vi "002_Data Source Manage.vi"(11 "Queue Ref In":T1={"UI"=refnum, "Message"=refnum, "Data"=refnum, "Caller"=refnum, "Name"="000 Common", "Data Path"=path "", "Class Path"=path "", "SubPanel"=refnum, "Project Name"="", "MNT"="", "Title"="", "Data Source"=refnum, "Queue List"={}, "VI"=refnum, "UE"=refnum}) -> ()   [LabVIEW 2020]
uses:
  Alin/QMH/000 Module Data Type.ctl
  Alin/QMH/Queue Message.ctl
  0007 Controls/002 Group Type.ctl
  0007 Controls/005 Data Source Type.ctl
  9999 SubVI/Global/Data Global/SDQ Data Type.ctl
  9999 SubVI/Global/Data Global/Data Global Mode.ctl
  <vilib>/Utility/file.llb/Read Delimited Spreadsheet (string).vi
  <vilib>/Utility/file.llb/Write Delimited Spreadsheet (string).vi
  <vilib>/Utility/config.llb/Write Key (String).vi
  <vilib>/Utility/config.llb/NI_LVConfig.lvlib
panel:
  in  "Module Launch":bool
  in  "Panel Show":bool
  in  "Data Source List":string(tree)
  out "Count":string
  in  "CAN Convert":bool
  in  "Show Info":bool
  in  "LabVIEW VISA":bool
  in  "SIEMENS S7":bool
  in  "FCTS DAQ":bool
  in  "Log List":i32(listbox)
  out "Write Time":u32(graph)
  out "Log":string
  out "Time":string
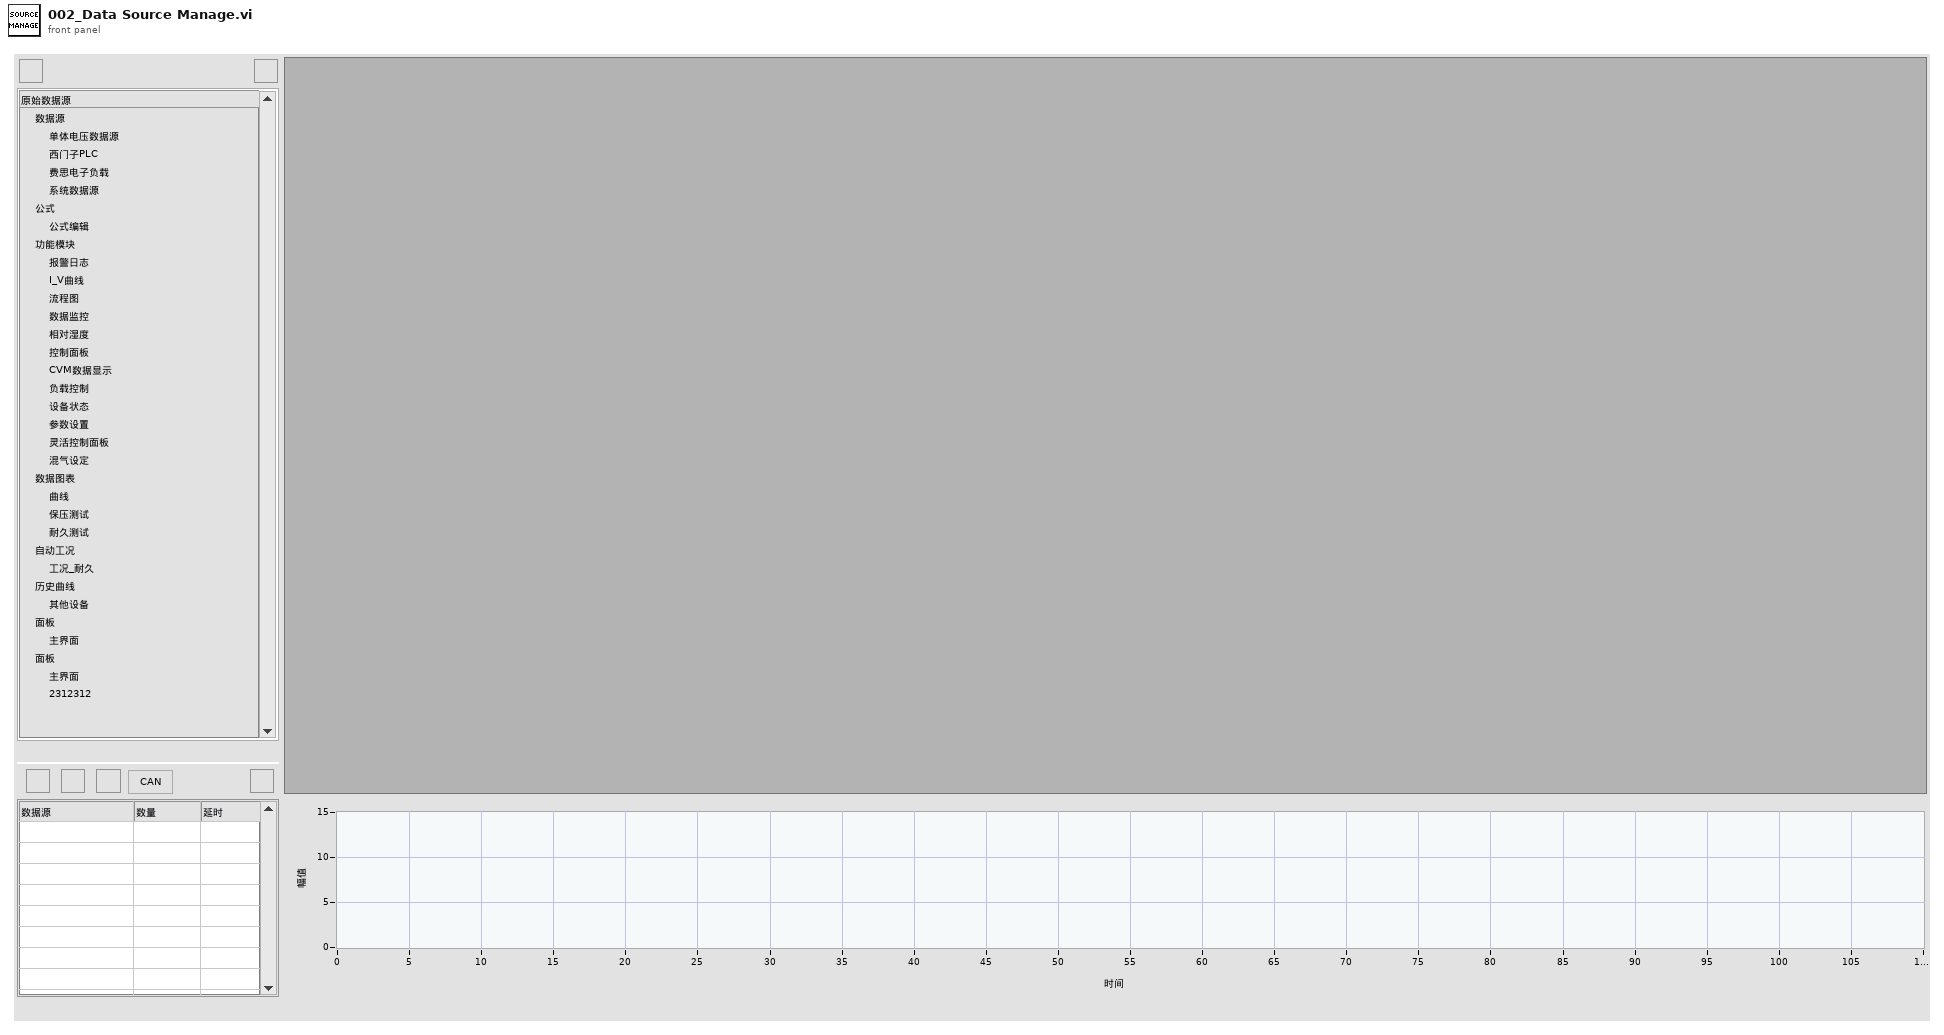
[diagram p1: front panel]
types:
  T1 = typedef "000 Module Data Type.ctl" = cluster{"UI":refnum<queue>, "Message":refnum<queue>, "Data":refnum<queue>, "Caller":refnum<queue>, "Name":string, "Data Path":path, "Class Path":path, "SubPanel":refnum<vi>, "Project Name":string, "MNT":string, "Title":string, "Data Source":refnum<queue>, "Queue List":map{string, refnum<queue>}, "VI":refnum<vi>, "UE":refnum<user-event>}
  T2 = typedef "SDQ Data Type.ctl" = cluster{"CAN Length":string, "CAN Name":string, "CAN ID":string, "CAN Type":string, "Test Item":string, "Byte Order":string, "Instruction":string, "Control Type":string, "Group":string, "Offset":dbl, "Coefficient":dbl, "Write Enable":bool, "Lable Type":string, "Key?":string, "Set Value":string, "Upper":dbl, "Lower":dbl, "Unit":string, "Formula":string, "Test Item Type":string, "Length":i32, "Address":string, "Name":string, "Identifier":string, "Data Type":string, "Enumerate?":string, "Enumerate List":string, "Data":string, "Source":string}
  T3 = cluster{"Queue":T1, "Source":map{string, map{string, T2}}, "All Data":map{string, T2}, "Type":cluster{"Name":string, "Data":map{string, T2}}, "Write Source":map{string, map{string, string}}, "Type":map{string, string}, "Log List":refnum<vi>, "Log":string[][], "Delay":cluster{"Count Time(ms)":u32, "Delay Time(ms)":u32, "Next":string}, "Internal?":bool, "Log Nane":string, "DataType":cluster{"Name":string, "Type":map{string, string}}, "DataMonitor":string[], "LoadControl":string}
  T4 = enum32{"Invalid", "Standard", "Closed", "Hidden", "Minimized", "Maximized"}
  T5 = typedef "Data Global Mode.ctl" = enum16{"Init", "Read", "Write", "Write Data", "Load"}
  T6 = cluster{"Name":string, "Type":map{string, string}}
  T7 = typedef "eventvkey.ctl" = enum16{"ASCII", "Enter", "Return", "Shift", "Ctrl", "Alt", "Cmd", "Opt", "Caps", "NumLock", "Clear", "Break", "Up", "Down", "Left", "Right", "Insert", "Delete", "Home", "End", "PageUp", "PageDown", "Escape", "Help", "Pause", "ScrollLock", "F1", "F2", "F3", "F4", "F5", "F6", "F7", "F8", "F9", "F10", "F11", "F12", "F13", "F14", "F15", "F16", "F17", "F18", "F19", "F20", "F21", "F22", "F23", "F24", "Play", "VolumeUp", "VolumeDown", "Mute", "Two Byte Char"}
  T8 = cluster{"Shift":bool, "Ctrl":bool, "Alt":bool, "Cmd":bool, "Opt":bool}
  T9 = typedef "002 Group Type.ctl" = cluster{"Name":string, "Enable":string, "Path":string}
  T10 = typedef "005 Data Source Type.ctl" = cluster{"Device Name":string, "Device Model":string, "Device Driver":string, "IP Address":string, "Port":string, "Remark":string, "Enable":string, "Path":string}
  T11 = cluster{"Queue":T1, "Data Source List":refnum<vi>, "SubPanel":refnum<vi>, "Group":cluster{"Group Title":string[], "Group Data":T9, "Group Name":string[]}, "Source":cluster{"Source Title":string[], "Source Data":T10, "Source Name":string[]}, "All Panel":string[], "GroupInfo":map{string, cluster{"Source":map{string, T10}, "Group":T9}}, "Class":map{string, cluster{"Device_Type":string, "Device_Manufacturer":string, "Driver":string, "Device_Model":string, "Class Path":path, "Defaule Config Path":string}}, "Version Path":path, "Source Launch?":bool, "Launch":bool}
  T12 = map{string, cluster{"Device_Type":string, "Device_Manufacturer":string, "Driver":string, "Device_Model":string, "Class Path":path, "Defaule Config Path":string}}
  T13 = cluster{"Device_Type":string, "Device_Manufacturer":string, "Driver":string, "Device_Model":string, "Class Path":path, "Defaule Config Path":string}
  T14 = map{string, cluster{"Source":map{string, T10}, "Group":T9}}
  T15 = cluster{"Data Out[0]":string, "Data Out[1]":string, "Data Out[2]":string}
  T16 = cluster{"[0]":string, "[1]":string, "[2]":string}
  T17 = cluster{"Data Out[0]":string, "Data Out[1]":string, "Data Out[2]":string, "Data Out[3]":string, "Data Out[4]":string, "Data Out[5]":string, "Data Out[6]":string, "Data Out[7]":string}
  T18 = cluster{"[0]":string, "[1]":string, "[2]":string, "[3]":string, "[4]":string, "[5]":string, "[6]":string, "[7]":string}
  T19 = typedef "NI_LVConfig.lvlib/Config Data RefNum.ctl" = refnum<k1>
  T20 = enum32{"invalid app kind", "Development System", "Run Time System", "Student Edition", "Embedded LabVIEW", "Evaluation", "Custom"}
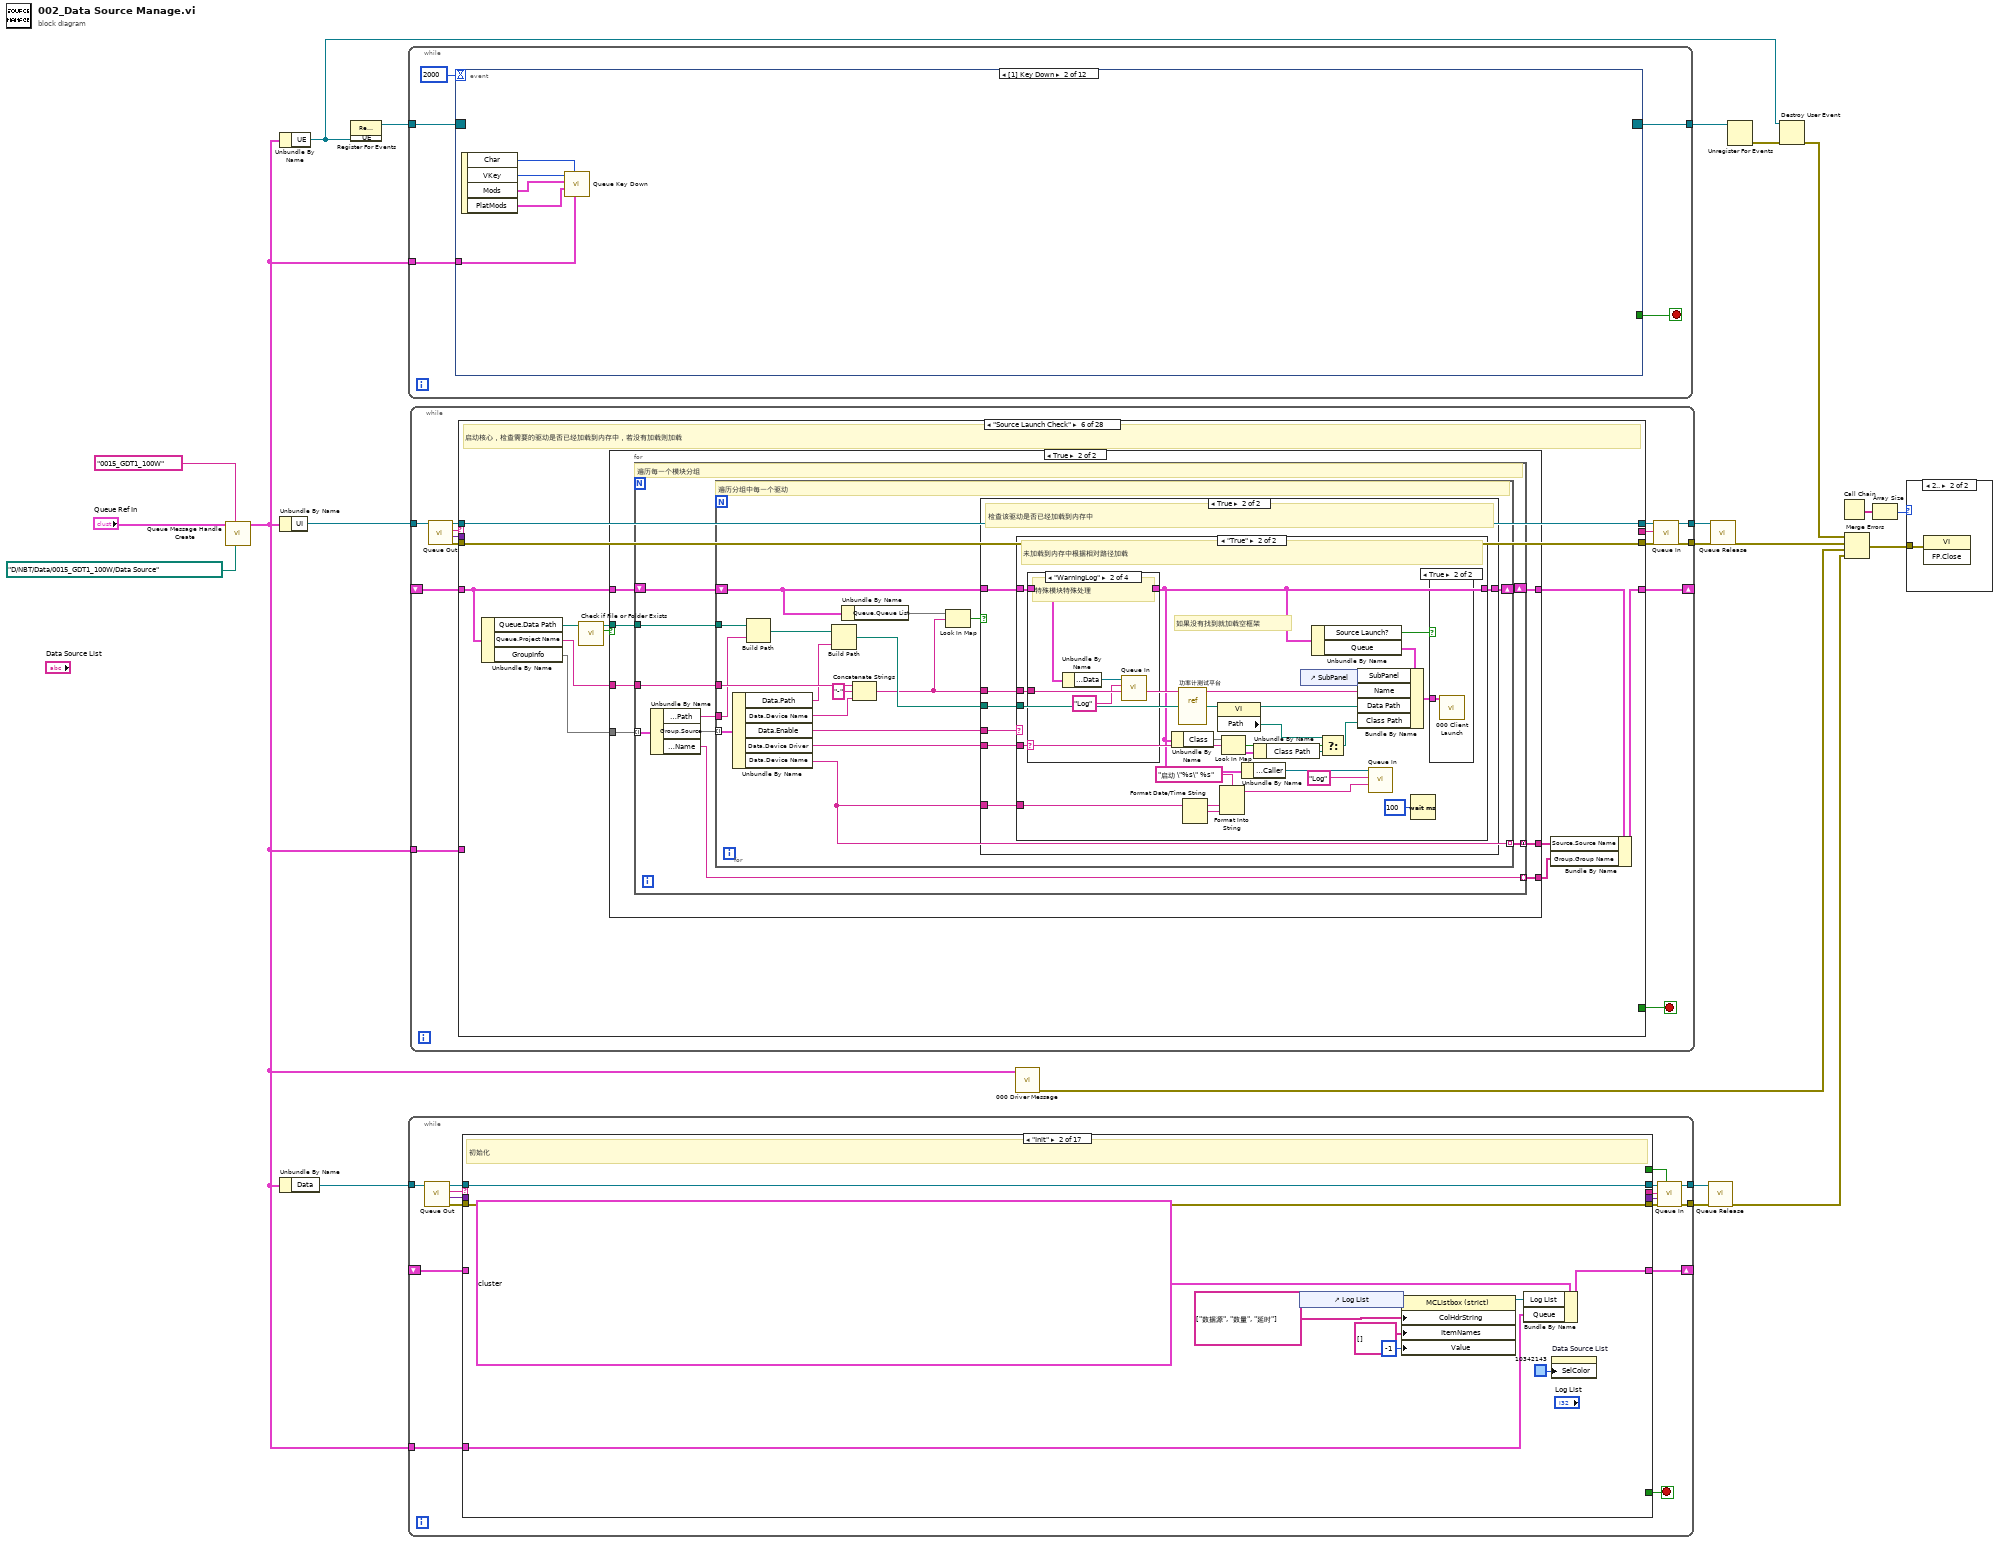
[diagram p0: block diagram]
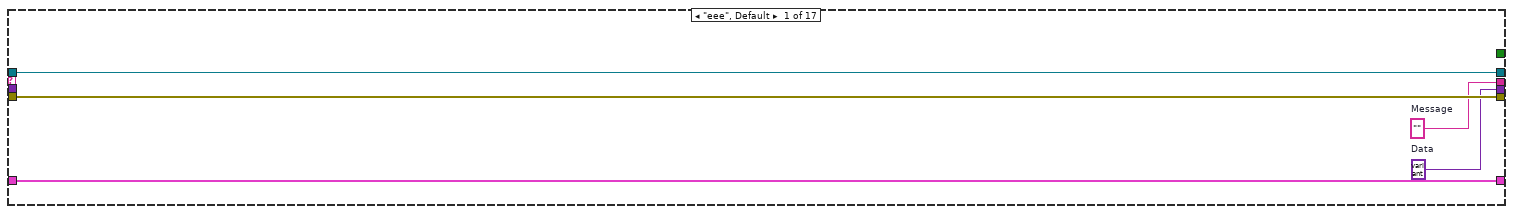
[diagram p2: hidden frame]
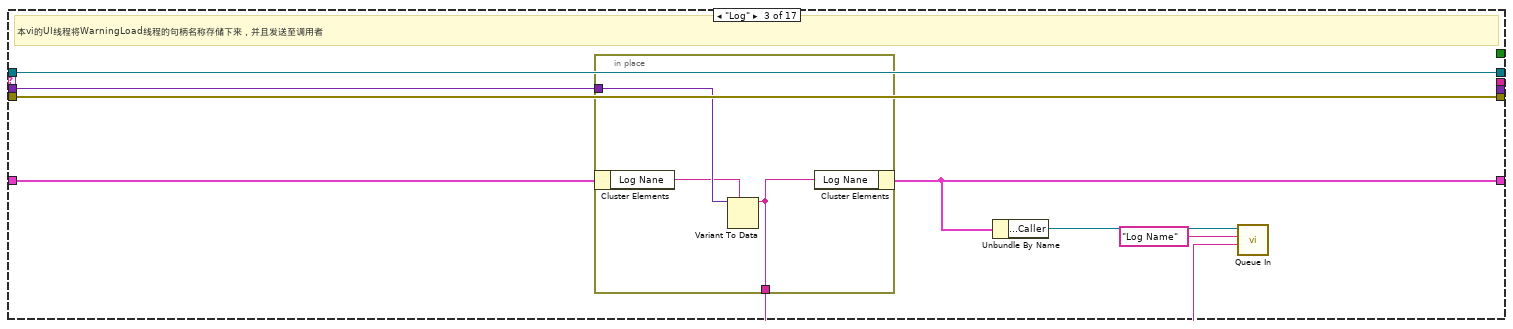
[diagram p3: hidden frame]
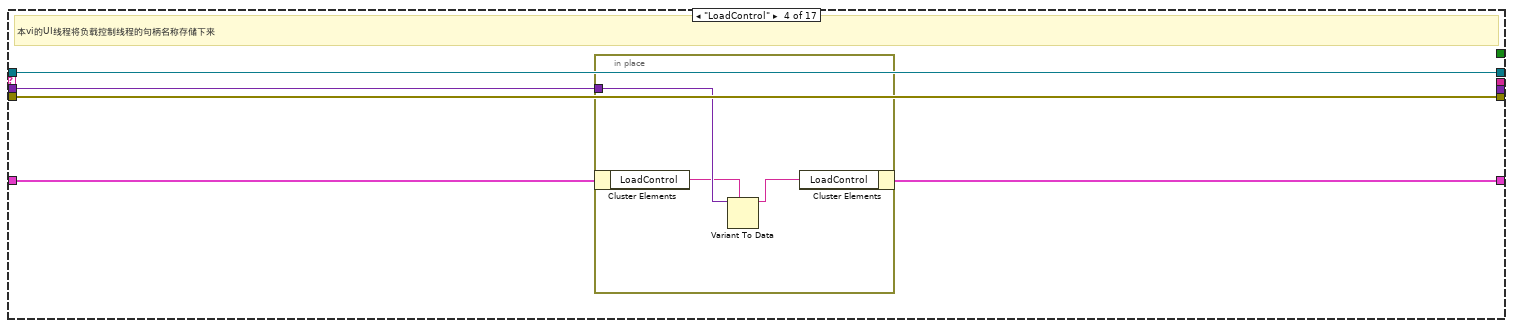
[diagram p4: hidden frame]
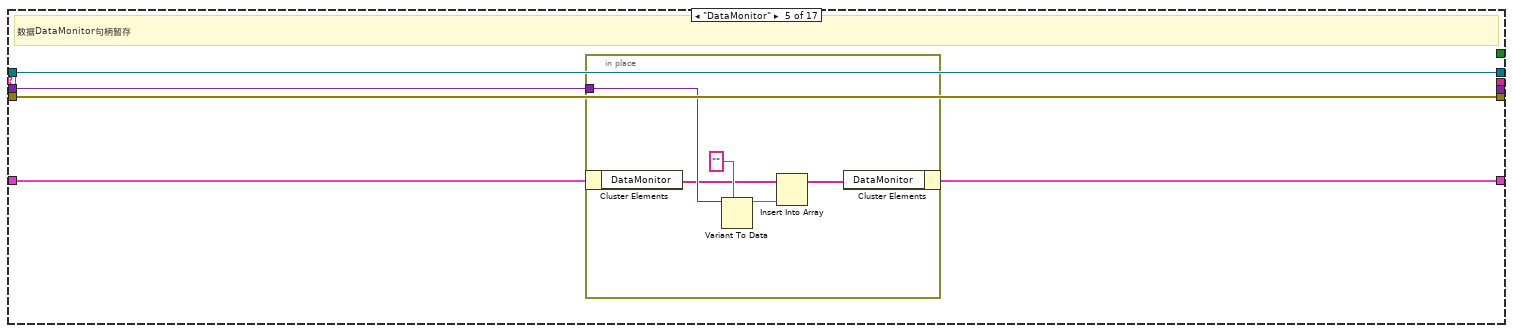
[diagram p5: hidden frame]
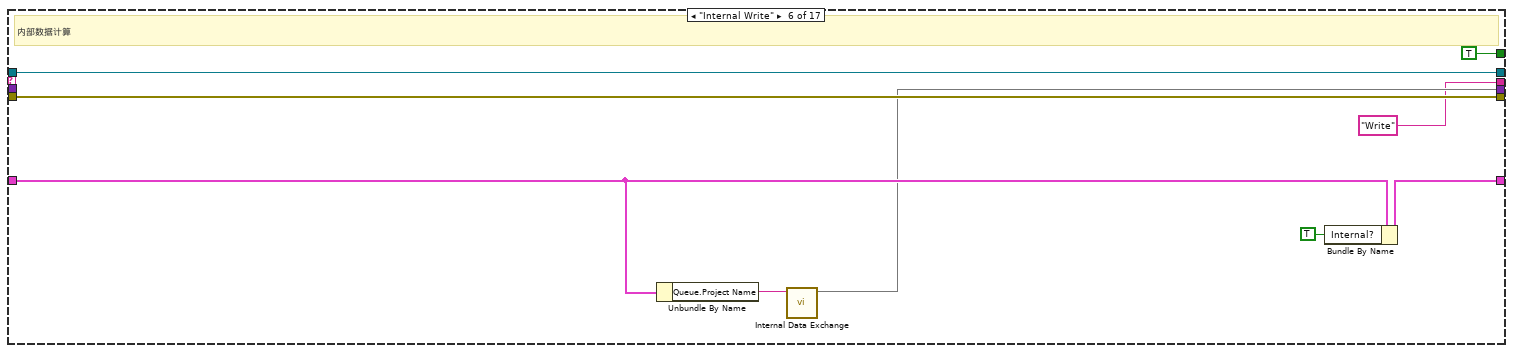
[diagram p6: hidden frame]
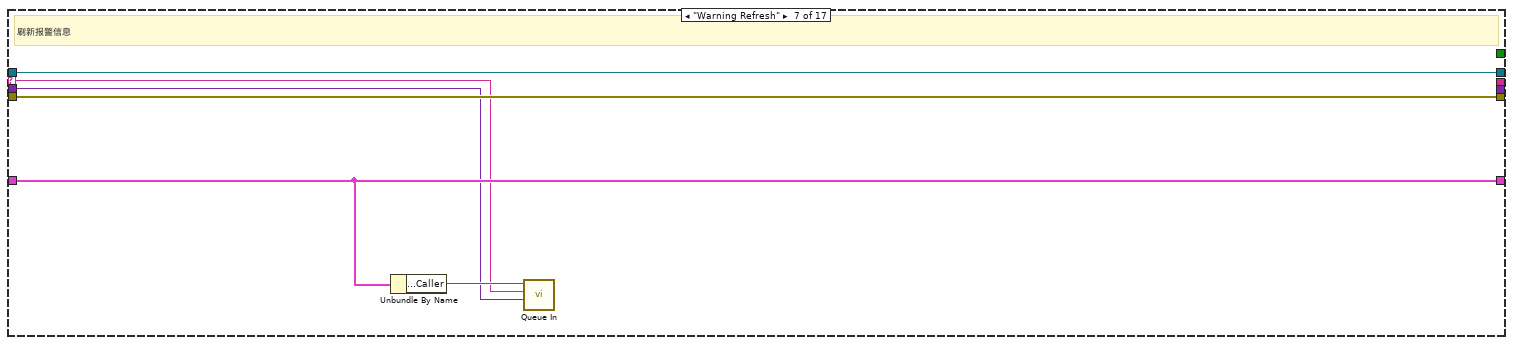
[diagram p7: hidden frame]
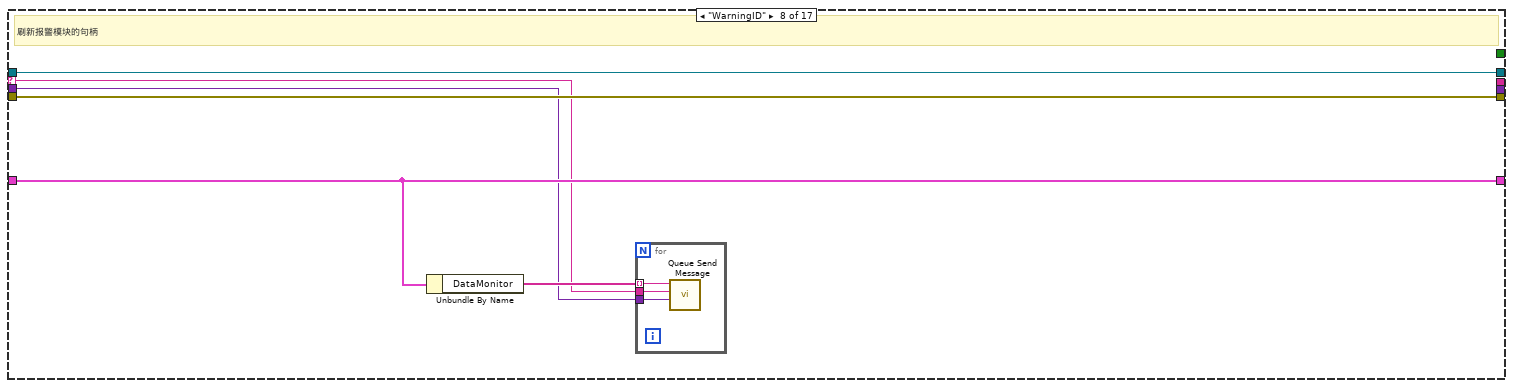
[diagram p8: hidden frame]
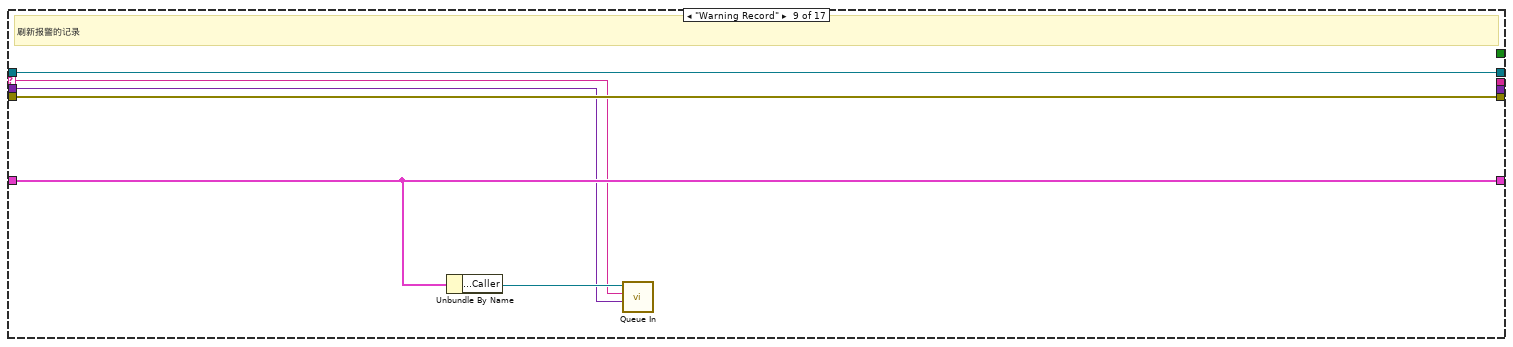
[diagram p9: hidden frame]
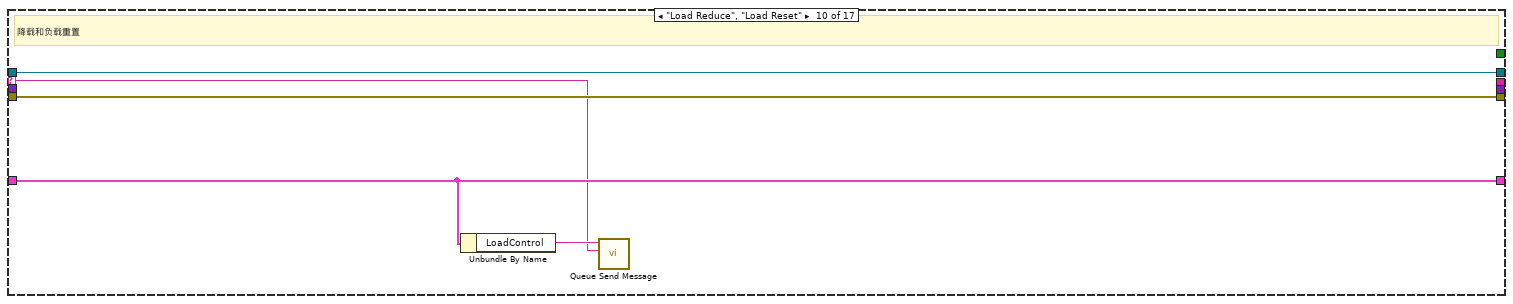
[diagram p10: hidden frame]
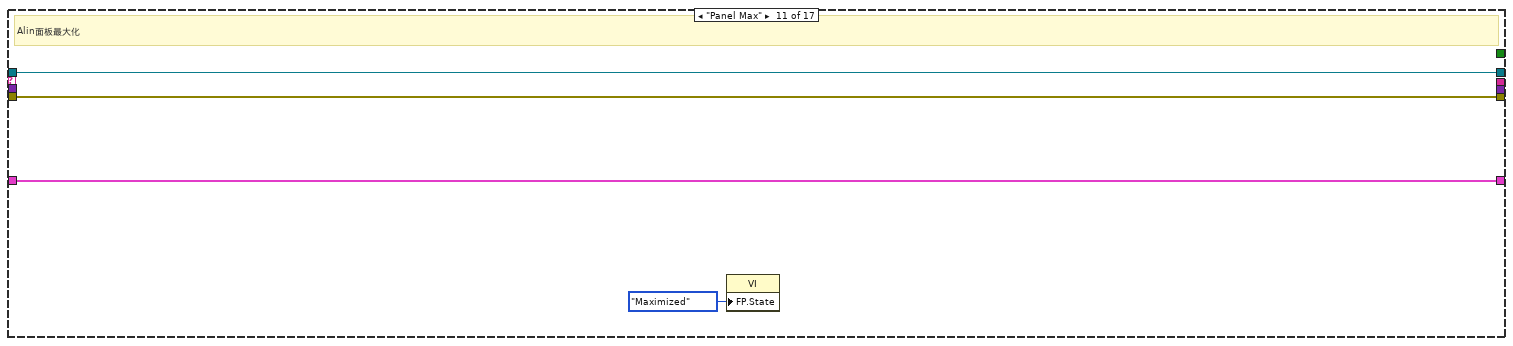
[diagram p11: hidden frame]
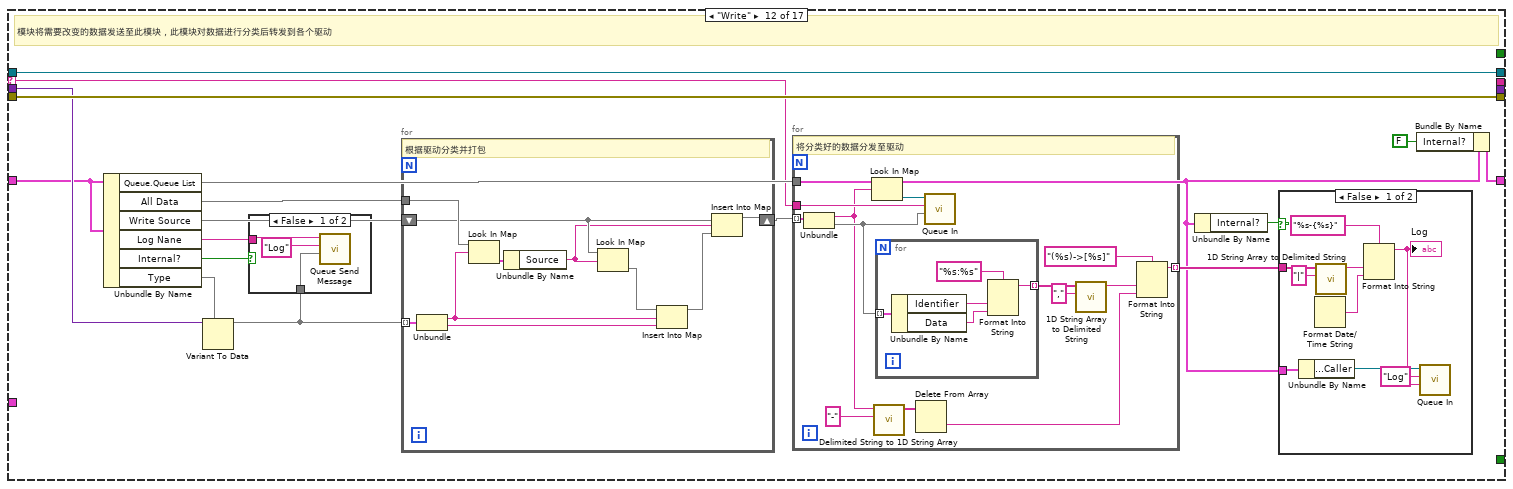
[diagram p12: hidden frame]
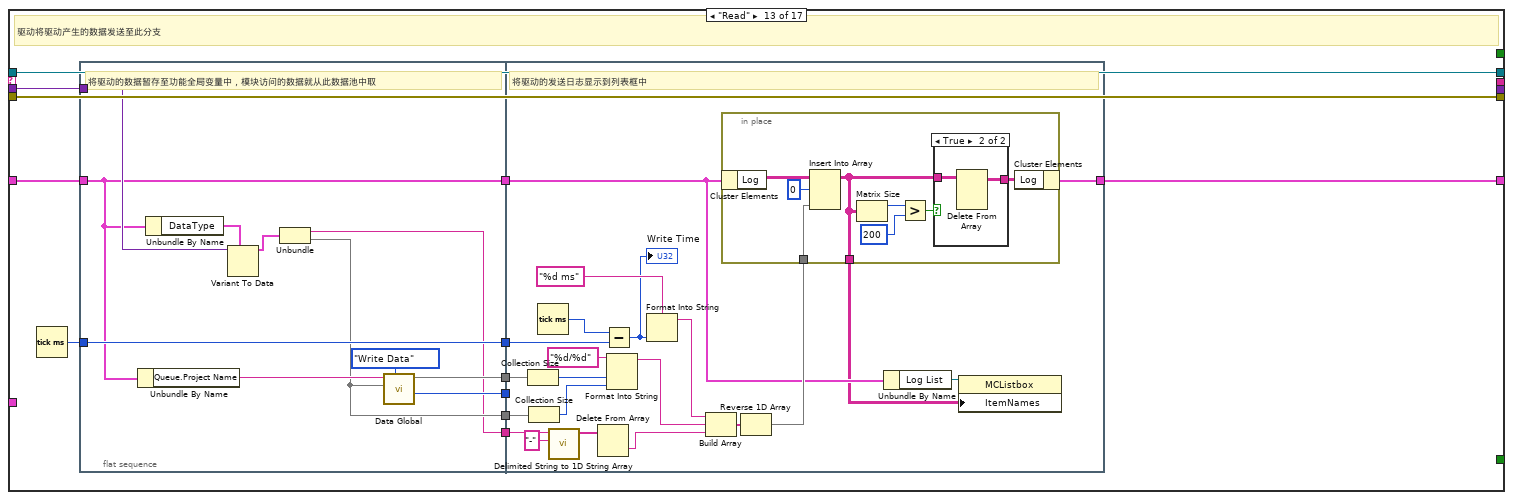
[diagram p15: hidden frame]
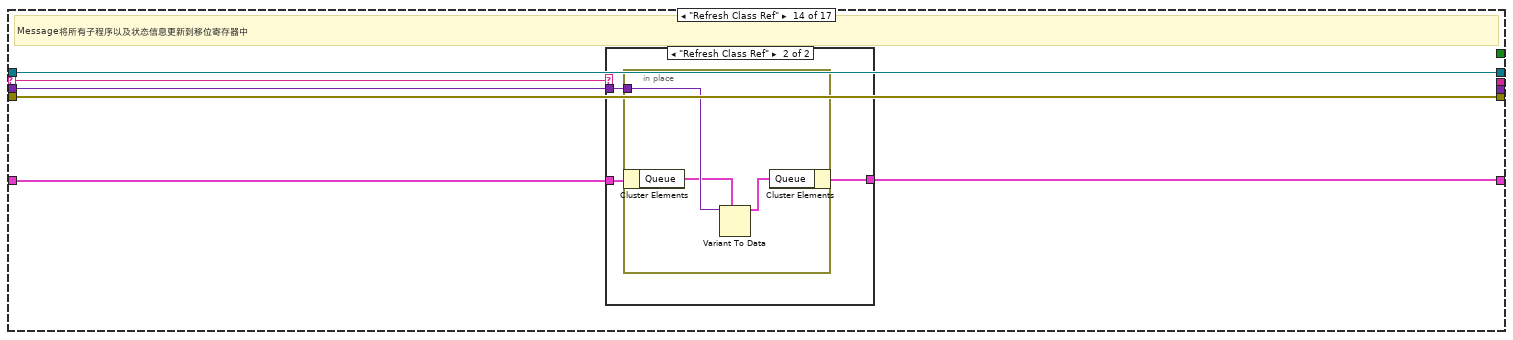
[diagram p17: hidden frame]
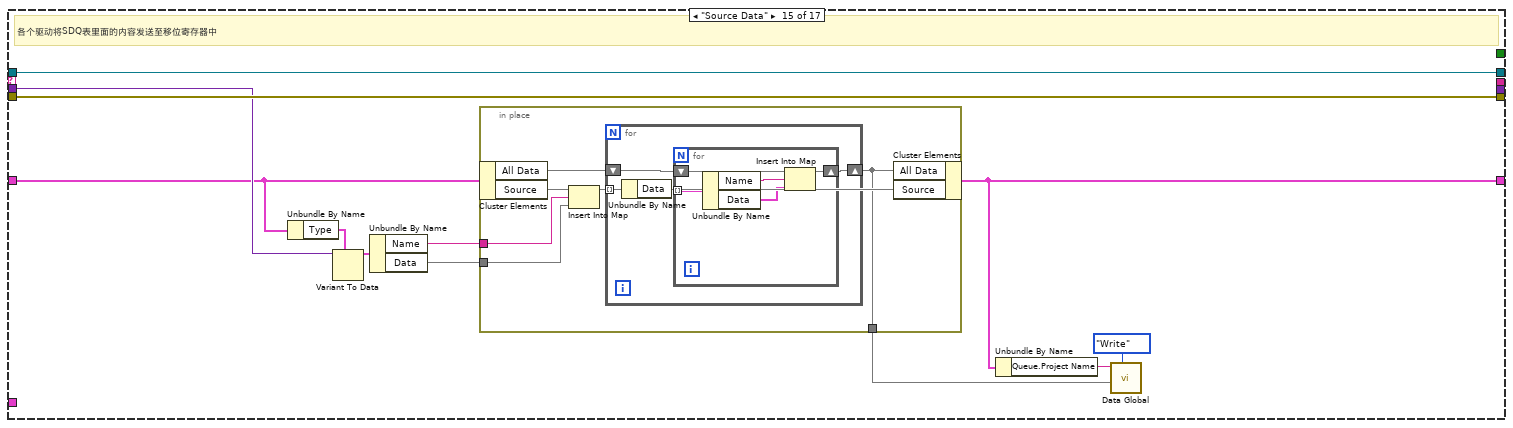
[diagram p19: hidden frame]
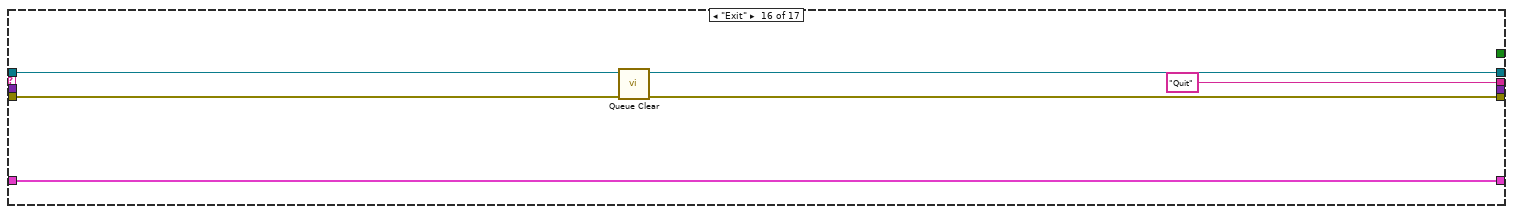
[diagram p20: hidden frame]
diagram:
  n1 = call "Queue Message Handle Create.vi"("Data Path"=path "D:/NBT/Data/0015_GDT1_100W/Data Source", "Project Name"="0015_GDT1_100W", "Queue Ref In"="Queue Ref In") -> ("Queue Ref Out"=w3:T1)  [unwired: 6 in, 2 out]
  n2 = Unbundle By Name(w3) -> ("UE"=w4:refnum<user-event>)
  n3 = Unbundle By Name(w3) -> ("UI"=w10:refnum<queue>)
  n4 = Unbundle By Name(w3) -> ("Data"=w18:refnum<queue>)
  n5 = register-events(w4) -> (reference out=w5:refnum<event-registration>)  [unwired: 2 in, 1 out]
  n6 = while {
    tunnel: w18 -> [w33]
    tunnel: [w30] -> w16
    tunnel: [w29] -> w17
    shift-right: [w25] -> _
    shift-left: _ -> [w24]
    tunnel: w3 -> [w22]
    stop <- w37 stop-if-true
    n7 = call "Queue Out.vi"("Queue In"=w33) -> ("error out"=w36:errorcluster, "Data"=w34:variant, "Message"=w35:string, "Queue Out"=w32:refnum<queue>)  [unwired: 6 in, 1 out]
    n8 = case shown="\"Init\"" w35 {
      selector: w35 -> [_ _ _ _ _ _ w93 w99 w108 w113 _ w130 _ w238 _ _ _]
      tunnel: w32 -> [w42 w53 w61 w69 w77 w91 w97 w103 w112 w117 w121 w138 w180 w240 w255 w279 w283]
      tunnel: w36 -> [w41 w52 w60 w68 w76 w90 w96 w102 w111 w116 w120 w137 w181 w239 w259 w277 w284]
      tunnel: [w42 w53 w61 w69 w77 w91 w97 w103 w112 w117 w121 w138 w180 w240 w255 w278 w283] -> w31
      tunnel: [w41 w52 w60 w68 w76 w90 w96 w102 w111 w116 w120 w137 w181 w239 w259 w276 w284] -> w28
      tunnel: [w40 _ _ _ _ "Write" ("Next") _ _ _ _ _ _ _ _ _ "Quit" _] -> w27
      tunnel: [_ _ _ _ _ _ _ _ _ _ _ _ _ _ _ _ TRUE] -> w37
      tunnel: [w39 _ _ _ _ w87 _ _ _ _ _ _ _ _ _ _ _] -> w26
      tunnel: w34 -> [_ _ w58 w66 w74 _ w92 w98 w107 _ _ w131 w189 w236 w258 _ _]
      tunnel: [w38 w49 w57 w65 w73 w86 w95 w101 w110 w115 w119 w123 w187 w235 w249 w275 w281] -> w25
      tunnel: w24 -> [w38 _ w59 w67 w75 w89 w95 w101 w110 w115 w119 w124 w188 w237 w257 w275 w281]
      tunnel: [_ _ _ _ _ TRUE _ _ _ _ _ _ _ _ _ _ _] -> w23
      tunnel: w22 -> [_ w43 _ _ _ _ _ _ _ _ _ _ _ _ _ _ _]
      frame "eee", Default {
        w39 = variant  # Data
        w40 = ""  # Message
      }
      frame "Init" {
        # "初始化"
        n9 = control-ref of="Log List"() -> (w48:refnum<vi>)
        n10 = property class="MCListbox (strict)"(reference=w48, "ColHdrString"=string[] ["数据源", "数量", "延时"] ("列首字符串[]"), "ItemNames"=string[][] [] ("项名"), "Value"=-1 ("值")) -> (reference out=w44:refnum<vi>)  [unwired: 1 in, 1 out]
        n11 = Bundle By Name(cluster=T3 {"Queue"={"UI"=refnum, "Message"=refnum, "Data"=refnum, "Caller"=refnum, "Name"="000 Common", "Data Path"=path "", "Class Path"=path "", "SubPanel"=refnum, "Project Name"="", "MNT"="", "Title"="", "Data Source"=refnum, "Queue List"={}, "VI"=refnum, "UE"=refnum}, "Source"={}, "All Data"={}, "Type"={"Name"="", "Data"={}}, "Write Source"={}, "Type"={}, "Log List"=refnum, "Log"=[], "Delay"={"Count Time(ms)"=5, "Delay Time(ms)"=1000, "Next"="Internal Write,Delay"}, "Internal?"=FALSE, "Log Nane"="", "DataType"={"Name"="", "Type"={}}, "DataMonitor"=[], "LoadControl"=""}, "Log List"=w44, "Queue"=w43) -> (w49:T3)
        n12 = property on="Data Source List" class="Tree (strict)"("SelColor"=u32 10342143 ("选择颜色")) -> ()  [unwired: 2 in, 2 out]
      }
      frame "Log" {
        # "本vi的UI线程将WarningLoad线程的句柄名称存储下来，并且发送至调用者"
        n13 = in-place {
          in-place-border: w58 -> [w64]
          in-place-border: [w62] -> w54
          n14 = in-place-cluster #1(w59) -> ("Log Nane"=w63:string)
          n15 = Variant To Data(type=w63, Variant=w64) -> (data=w62:string)  [unwired: 1 in, 1 out]
          n16 = in-place-cluster #1("Log Nane"=w62) -> (w57:T3)
        }
        n17 = Unbundle By Name(w57) -> ("Queue.Caller"=w56:refnum<queue>)
        n18 = call "Queue In.vi"("Data"=w54, "Message"="Log Name", "Queue In"=w56) -> ()  [unwired: 7 in, 2 out]
      }
      frame "LoadControl" {
        # "本vi的UI线程将负载控制线程的句柄名称存储下来"
        n19 = in-place {
          in-place-border: w66 -> [w72]
          n20 = in-place-cluster #2(w67) -> ("LoadControl"=w71:string)
          n21 = Variant To Data(type=w71, Variant=w72) -> (data=w70:string)  [unwired: 1 in, 1 out]
          n22 = in-place-cluster #2("LoadControl"=w70) -> (w65:T3)
        }
      }
      frame "DataMonitor" {
        # "数据DataMonitor句柄暂存"
        n23 = in-place {
          in-place-border: w74 -> [w82]
          n24 = in-place-cluster #3(w75) -> ("DataMonitor"=w80:string[])
          n25 = Variant To Data(type="", Variant=w82) -> (data=w79:string)  [unwired: 1 in, 1 out]
          n26 = Insert Into Array(array=w80, new element=w79) -> (w78:string[])  [unwired: 1 in]
          n27 = in-place-cluster #3("DataMonitor"=w78) -> (w73:T3)
        }
      }
      frame "Internal Write" {
        # "内部数据计算"
        n28 = Unbundle By Name(w89) -> ("Queue.Project Name"=w88:string)
        n29 = call "Internal Data Exchange.vi"("Project"=w88) -> ("Write Data"=w87:map{string, string})  [unwired: 9 in, 1 out]
        n30 = Bundle By Name(cluster=w89, "Internal?"=TRUE) -> (w86:T3)
      }
      frame "Warning Refresh" {
        # "刷新报警信息"
        n31 = Unbundle By Name(w95) -> ("Queue.Caller"=w94:refnum<queue>)
        n32 = call "Queue In.vi"("Data"=w92, "Message"=w93, "Queue In"=w94) -> ()  [unwired: 7 in, 2 out]
      }
      frame "WarningID" {
        # "刷新报警模块的句柄"
        n33 = Unbundle By Name(w101) -> ("DataMonitor"=w100:string[])
        n34 = for {
          tunnel: w100 -> [w106] mode=indexing
          tunnel: w99 -> [w105]
          tunnel: w98 -> [w104]
          n35 = call "Queue Send Message.vi"("Data"=w104, "Message"=w105, "Queue Name"=w106) -> ()  [unwired: 6 in, 3 out]
        }
      }
      frame "Warning Record" {
        # "刷新报警的记录"
        n36 = Unbundle By Name(w110) -> ("Queue.Caller"=w109:refnum<queue>)
        n37 = call "Queue In.vi"("Data"=w107, "Message"=w108, "Queue In"=w109) -> ()  [unwired: 7 in, 2 out]
      }
      frame "Load Reduce", "Load Reset" {
        # "降载和负载重置"
        n38 = Unbundle By Name(w115) -> ("LoadControl"=w114:string)
        n39 = call "Queue Send Message.vi"("Message"=w113, "Queue Name"=w114) -> ()  [unwired: 7 in, 3 out]
      }
      frame "Panel Max" {
        # "Alin面板最大化"
        n40 = property class="VI"("FP.State"=T4."Maximized" ("前面板窗口:状态")) -> ()  [unwired: 2 in, 2 out]
      }
      frame "Write" {
        # "模块将需要改变的数据发送至此模块，此模块对数据进行分类后转发到各个驱动"
        n41 = Unbundle By Name(w124) -> ("Queue.Queue List"=w136:map{string, refnum<queue>}, "All Data"=w134:map{string, T2}, "Write Source"=w135:map{string, map{string, string}}, "Log Nane"=w132:string, "Internal?"=w127:bool, "Type"=w125:map{string, string})
        n42 = Variant To Data(type=w125, Variant=w131) -> (data=w129:map{string, string})  [unwired: 1 in, 1 out]
        n43 = case shown="False" w127 {
          tunnel: w132 -> [w150 _]
          tunnel: w129 -> [w148 _]
          frame False {
            n44 = call "Queue Send Message.vi"("Data"=w148, "Message"="Log", "Queue Name"=w150) -> ()  [unwired: 6 in, 3 out]
          }
          frame True {
          }
        }
        n45 = for {
          shift-right: [w175] -> w133
          shift-left: w135 -> [w176]
          tunnel: w129 -> [w170] mode=indexing
          tunnel: w134 -> [w178]
          # "根据驱动分类并打包"
          n46 = Unbundle(w170) -> ("Identifier"=w172:string, "Data"=w171:string)
          n47 = Look In Map(map=w178, key=w172) -> (value=w179:T2)  [unwired: 1 in, 1 out]
          n48 = Unbundle By Name(w179) -> ("Source"=w173:string)
          n49 = Look In Map(map=w176, key=w173) -> (value=w177:map{string, string})  [unwired: 1 in, 1 out]
          n50 = Insert Into Map(map in=w177, key=w172, value=w171) -> (map out=w174:map{string, string})  [unwired: 2 out]
          n51 = Insert Into Map(map in=w176, key=w173, value=w174) -> (map out=w175:map{string, map{string, string}})  [unwired: 2 out]
        }
        n52 = for {
          tunnel: w136 -> [w164]
          tunnel: w130 -> [w163]
          tunnel: w133 -> [w161] mode=indexing
          tunnel: [w155] -> w128 mode=indexing
          # "将分类好的数据分发至驱动"
          n53 = Unbundle(w161) -> ("Source"=w154:string, "Write"=w160:map{string, string})
          n54 = Look In Map(map=w164, key=w154) -> (value=w162:refnum<queue>)  [unwired: 1 in, 1 out]
          n55 = call <vilib>:"Delimited String to 1D String Array.vi"("delimiter"="-", "delimited string"=w154) -> ("string array"=w152:string[])  [unwired: 9 in]
          n56 = for {
            tunnel: w160 -> [w169] mode=indexing
            tunnel: [w165] -> w156 mode=indexing
            n57 = Unbundle By Name(w169) -> ("Identifier"=w167:string, "Data"=w166:string)
            n58 = Format Into String(format string="%s:%s" ("格式字符串"), w167, w166) -> (resulting string=w165:string)  [unwired: 2 in, 1 out]
          }
          n59 = Delete From Array(array=w152) -> (deleted portion=w151:string)  [unwired: 2 in, 1 out]
          n60 = call "Queue In.vi"("Data"=w160, "Message"=w163, "Queue In"=w162) -> ()  [unwired: 7 in, 2 out]
          n61 = call <vilib>:"1D String Array to Delimited String.vi"("delimiter"=",", "string array"=w156) -> ("delimited string"=w159:string)  [unwired: 9 in]
          n62 = Format Into String(format string="(%s)->[%s]" ("格式字符串"), w159, w151) -> (resulting string=w155:string)  [unwired: 2 in, 1 out]
        }
        n63 = Unbundle By Name(w124) -> ("Internal?"=w126:bool)
        n64 = case shown="False" w126 {
          tunnel: w128 -> [w146 _]
          tunnel: w124 -> [w142 _]
          frame False {
            n65 = Unbundle By Name(w142) -> ("Queue.Caller"=w141:refnum<queue>)
            n66 = Format Date/Time String() -> (date/time string=w145:string)  [unwired: 3 in]
            n67 = call <vilib>:"1D String Array to Delimited String.vi"("delimiter"="|", "string array"=w146) -> ("delimited string"=w144:string)  [unwired: 9 in]
            n68 = Format Into String(format string="%s-{%s}" ("格式字符串"), w144, w145) -> (resulting string=w140:string)  [unwired: 2 in, 1 out]
            "Log" <- w140
            n69 = call "Queue In.vi"("Data"=w140, "Message"="Log", "Queue In"=w141) -> ()  [unwired: 7 in, 2 out]
          }
          frame True {
          }
        }
        n70 = Bundle By Name(cluster=w124, "Internal?"=FALSE) -> (w123:T3)
      }
      frame "Read" {
        # "驱动将驱动产生的数据发送至此分支"
        n71 = Tick Count (ms)() -> (millisecond timer value=w186:u32)
        n72 = flat-sequence {
          tunnel: w189 -> [w202]
          tunnel: w188 -> [w195]
          tunnel: [w195] -> w191
          tunnel: w186 -> [w200]
          tunnel: [w200] -> w190
          tunnel: [w198] -> w185
          tunnel: [w197] -> w184
          tunnel: [w192] -> w183
          tunnel: [w193] -> w182
          tunnel: [w215] -> w187
          tunnel: w191 -> [w213]
          tunnel: w190 -> [w222]
          tunnel: w185 -> [w221]
          tunnel: w184 -> [_]
          tunnel: w183 -> [w209]
          tunnel: w182 -> [w205]
          frame #0 {
            # "将驱动的数据暂存至功能全局变量中，模块访问的数据就从此数据池中取"
            n73 = Unbundle By Name(w195) -> ("Queue.Project Name"=w199:string)
            n74 = Unbundle By Name(w195) -> ("DataType"=w201:T6)
            n75 = Variant To Data(type=w201, Variant=w202) -> (data=w194:T6)  [unwired: 1 in, 1 out]
            n76 = Unbundle(w194) -> ("Name"=w192:string, "Type"=w193:map{string, string})
            n77 = call "Data Global.vi"("Operate"=Data_Global_Mode."Write Data", "Data"=w193, "Name"=w199) -> ("x-y"=w197:u32, "Data Out"=w198:map{string, T2})  [unwired: 5 in, 2 out]
          }
          frame #1 {
            # "将驱动的发送日志显示到列表框中"
            n78 = Collection Size(1:w221) -> (0:w211:i32)
            n79 = Collection Size(1:w205) -> (0:w204:i32)
            n80 = Tick Count (ms)() -> (millisecond timer value=w223:u32)
            n81 = call <vilib>:"Delimited String to 1D String Array.vi"("delimiter"="-", "delimited string"=w209) -> ("string array"=w207:string[])  [unwired: 9 in]
            n82 = Delete From Array(array=w207) -> (deleted portion=w206:string)  [unwired: 2 in, 1 out]
            n83 = Subtract(x=w223, y=w222) -> (x-y=w203:u32)
            "Write Time" <- w203
            n84 = Format Into String(format string="%d/%d" ("格式字符串"), w211, w204) -> (resulting string=w217:string)  [unwired: 2 in, 1 out]
            n85 = Format Into String(format string="%d ms" ("格式字符串"), w203) -> (resulting string=w218:string)  [unwired: 2 in, 1 out]
            n86 = Build Array(w218, w217, w206) -> (w216:string[])
            n87 = Reverse 1D Array(array=w216) -> (reversed array=w214:string[])
            n88 = in-place {
              in-place-border: w214 -> [w229]
              in-place-border: [w224] -> w212
              n89 = in-place-cluster #4(w213) -> ("Log"=w231:string[][])
              n90 = Insert Into Array(array=w231, index (row)=0 ("索引 (行)"), new element=w229) -> (w224:string[][])  [unwired: 1 in]
              n91 = Matrix Size(0:w224) -> (1:w228:i32)  [unwired: 1 out]
              n92 = Greater?(x=w228, y=200) -> (0:w226:bool)
              n93 = case shown="True" w226 {
                tunnel: w224 -> [w232 w234]
                tunnel: [w232 w233] -> w225
                frame False {
                }
                frame True {
                  n94 = Delete From Array(array=w234) -> (array with subset deleted=w233:string[][])  [unwired: 3 in, 1 out]
                }
              }
              n95 = in-place-cluster #4("Log"=w225) -> (w215:T3)
            }
            n96 = Unbundle By Name(w213) -> ("Log List"=w210:refnum<vi>)
            n97 = property class="MCListbox"(reference=w210, "ItemNames"=w212) -> ()  [unwired: 1 in, 2 out]
          }
        }
      }
      frame "Refresh Class Ref" {
        # "Message将所有子程序以及状态信息更新到移位寄存器中"
        n98 = case shown="\"Refresh Class Ref\"" w238 {
          tunnel: w237 -> [w241 w244]
          tunnel: w236 -> [_ w243]
          tunnel: [w241 w242] -> w235
          frame "eee", Default {
          }
          frame "Refresh Class Ref" {
            n99 = in-place {
              in-place-border: w243 -> [w247]
              n100 = in-place-cluster #5(w244) -> ("Queue"=w246:T1)
              n101 = Variant To Data(type=w246, Variant=w247) -> (data=w245:T1)  [unwired: 1 in, 1 out]
              n102 = in-place-cluster #5("Queue"=w245) -> (w242:T3)
            }
          }
        }
      }
      frame "Source Data" {
        # "各个驱动将SDQ表里面的内容发送至移位寄存器中"
        n103 = Unbundle By Name(w257) -> ("Type"=w252:cluster{"Name":string, "Data":map{string, T2}})
        n104 = Variant To Data(type=w252, Variant=w258) -> (data=w254:cluster{"Name":string, "Data":map{string, T2}})  [unwired: 1 in, 1 out]
        n105 = Unbundle By Name(w254) -> ("Name"=w253:string, "Data"=w256:map{string, T2})
        n106 = in-place {
          in-place-border: w253 -> [w261]
          in-place-border: w256 -> [w262]
          in-place-border: [w260] -> w250
          n107 = in-place-cluster #6(w257) -> ("All Data"=w264:map{string, T2}, "Source"=w265:map{string, map{string, T2}})
          n108 = Insert Into Map(map in=w265, key=w261, value=w262) -> (map out=w263:map{string, map{string, T2}})  [unwired: 2 out]
          n109 = for {
            shift-right: [w268] -> w260
            shift-left: w264 -> [w269]
            tunnel: w263 -> [w267] mode=indexing
            n110 = Unbundle By Name(w267) -> ("Data"=w266:map{string, T2})
            n111 = for {
              tunnel: w266 -> [w272] mode=indexing
              shift-right: [w273] -> w268
              shift-left: w269 -> [w274]
              n112 = Unbundle By Name(w272) -> ("Name"=w271:string, "Data"=w270:T2)
              n113 = Insert Into Map(map in=w274, key=w271, value=w270) -> (map out=w273:map{string, T2})  [unwired: 2 out]
            }
          }
          n114 = in-place-cluster #6("All Data"=w260, "Source"=w263) -> (w249:T3)
        }
        n115 = Unbundle By Name(w249) -> ("Queue.Project Name"=w248:string)
        n116 = call "Data Global.vi"("Operate"=Data_Global_Mode."Write", "Data In"=w250, "Name"=w248) -> ()  [unwired: 5 in, 4 out]
      }
      frame "Exit" {
        n117 = call "Queue Clear.vi"("error in (no error)"=w277, "Queue In"=w279) -> ("error out"=w276:errorcluster, "Queue Out"=w278:refnum<queue>)  [unwired: 8 in]
      }
      frame "Quit" {
      }
    }
    n118 = call "Queue In.vi"("First"=w23, "error in (no error)"=w28, "Data"=w26, "Message"=w27, "Queue In"=w31) -> ("error out"=w29:errorcluster, "Queue Out"=w30:refnum<queue>)  [unwired: 5 in]
  }
  n119 = while {
    tunnel: w5 -> [w289]
    tunnel: [w287] -> w6
    tunnel: w3 -> [w286]
    stop <- w288 stop-if-true
    n120 = event shown="[1] Key Down" {
      selector: w289 -> [_ _ _ _ _ _ _ _ _ _ _ _]
      dyn-events: [_ _ _ _ _ _ _ _ _ _ _ _] -> w287
      timeout: 2000 -> [_ _ _ _ _ _ _ _ _ _ _ _]
      tunnel: [_ _ _ _ _ _ w343 _ _ _ _ _] -> w288
      tunnel: w286 -> [w292 w294 _ _ w338 w342 _ w351 w368 w377 _ w426]
      event Timeout {
        n121 = event-data() -> ()  [unwired: 1 in, 1 out]
        n122 = Unbundle By Name(w292) -> ("Data"=w291:refnum<queue>)
        n123 = call "Queue In.vi"("Message"="Internal Write", "Queue In"=w291) -> ()  [unwired: 8 in, 2 out]
        n124 = Format Date/Time String() -> (date/time string=→"Time":string)  [unwired: 3 in]
      }
      event Key Down {
        n125 = event-data() -> ("Char"=w297:i16, "VKey"=w298:T7, "Mods"=w296:cluster{"Num Pad":bool, "Menu Key":bool}, "PlatMods"=w295:T8)  [unwired: 1 in]
        n126 = call "Queue Key Down.vi"("Queue Ref Out"=w294, "C"=w297, "Platform Key"=w295, "Group Key"=w296, "V Key"=w298) -> ()  [unwired: 6 in, 1 out]
      }
      event "Time": Mouse Down {
        n127 = event-data() -> ("Mods.Double Click"=w299:bool)  [unwired: 1 in]
        n128 = case shown="True" w299 {
          frame False {
          }
          frame True {
            n129 = vi-ref "Queue Number Check.vi"() -> (w300:refnum<vi>)
            n130 = property class="VI"(reference=w300) -> (reference out=w302:refnum<vi>, "Path"=w301:path)  [unwired: 1 in, 1 out]
            n131 = property class="VI"(reference=w302) -> ("FP.State"=w303:T4)  [unwired: 1 in, 2 out]
            n132 = case shown="\"Invalid\", Default" w303 {
              tunnel: w301 -> [w310 _]
              frame "Invalid", Default {
                n133 = Open VI Reference(vi path=w310) -> (vi reference=w309:refnum<vi>)  [unwired: 5 in, 1 out]
                n134 = invoke class="VI" method="FP.Open"(reference=w309, "Activate"=TRUE ("激活？"), "State"=T4."Standard" ("状态")) -> (reference out=w306:refnum<vi>)  [unwired: 2 in, 4 out]
                n135 = invoke class="VI" method="Run VI"(reference=w306, "Wait until done"=FALSE ("结束前等待"), "Auto Dispose Ref"=TRUE ("自动销毁引用")) -> ()  [unwired: 2 in, 5 out]
              }
              frame "Standard" {
              }
            }
          }
        }
      }
      event "Show Info": Value Change {
        n136 = event-data() -> ("NewVal"=w312:bool)  [unwired: 1 in]
        n137 = flat-sequence {
          tunnel: w312 -> [w319]
          tunnel: [w313] -> w311
          tunnel: w311 -> [w323]
          frame #0 {
            n138 = case shown="True" w319 {
              selector: w319 -> [_ w322]
              tunnel: [_ w322] -> w313
              tunnel: [4 200] -> w315
              frame False {
              }
              frame True {
              }
            }
            n139 = property on="Write Time" class="WFChart (strict)"("Visible"=w313) -> ()  [unwired: 2 in, 2 out]
            n140 = property on="Log List" class="MCListbox (strict)"("Visible"=w313) -> ()  [unwired: 2 in, 2 out]
            n141 = control-ref of="分隔栏 2"() -> (w318:refnum<vi>)
            n142 = property class="Splitter"(reference=w318) -> ("Position"=w316:i32)  [unwired: 1 in, 2 out]
            n143 = control-ref of="分隔栏 3"() -> (w317:refnum<vi>)
            n144 = Subtract(x=w316, y=w315) -> (x-y=w314:i32)
            n145 = property class="Splitter"(reference=w317, "Position"=w314) -> ()  [unwired: 1 in, 2 out]
          }
          frame #1 {
            n146 = case shown="True" w323 {
              frame False {
              }
              frame True {
                n147 = control-ref of="Write Time"() -> (w335:refnum<vi>)
                n148 = control-ref of="Log List"() -> (w331:refnum<vi>)
                n149 = property class="WFChart (严格)"(reference=w335) -> (reference out=w333:refnum<vi>, "OwningPane"=w332:refnum<vi>)  [unwired: 1 in, 1 out]
                n150 = property class="MCListbox (严格)"(reference=w331) -> (reference out=w329:refnum<vi>, "OwningPane"=w330:refnum<vi>)  [unwired: 1 in, 1 out]
                n151 = property class="Pane"(reference=w332) -> ("Height"=w325:u32, "Width"=w334:u32)  [unwired: 1 in, 2 out]
                n152 = property class="Pane"(reference=w330) -> ("Height"=w327:u32, "Width"=w328:u32)  [unwired: 1 in, 2 out]
                n153 = expression code="x-60"(w334) -> (w326:u32)
                n154 = expression code="x-60"(w325) -> (w324:u32)
                n155 = property class="MCListbox (严格)"(reference=w329, "Height"=w327, "Width"=w328) -> ()  [unwired: 1 in, 2 out]
                n156 = property class="WFChart (严格)"(reference=w333, "Height"=w324, "Width"=w326) -> ()  [unwired: 1 in, 2 out]
              }
            }
          }
        }
      }
      event "FCTS DAQ", "SIEMENS S7", "LabVIEW VISA", "Panel Show", "Module Launch", "CAN Convert": Value Change {
        n157 = event-data() -> ("CtlRef"=w339:refnum<vi>)  [unwired: 1 in]
        n158 = Unbundle By Name(w338) -> ("UI"=w337:refnum<queue>)
        n159 = property class="Bool"(reference=w339) -> ("Label.Text"=w336:string)  [unwired: 1 in, 2 out]
        n160 = call "Queue In.vi"("Message"=w336, "Queue In"=w337) -> ()  [unwired: 8 in, 2 out]
      }
      event Panel Resize {
        n161 = event-data() -> ()  [unwired: 1 in, 1 out]
        n162 = Unbundle By Name(w342) -> ("Message"=w341:refnum<queue>)
        n163 = call "Queue In.vi"("Message"="Panel Change", "Queue In"=w341) -> ()  [unwired: 8 in, 2 out]
      }
      event User Event {
        n164 = event-data() -> ("Message"=w345:string)  [unwired: 1 in]
        n165 = Equal?(x=w345, y="Exit") -> (x = y?=w343:bool)
      }
      event Panel Close? {
        n166 = event-data() -> ()  [unwired: 1 in, 1 out]
        n167 = Call Chain() -> (call chain=w350:string[])
        n168 = Array Size(array=w350) -> (size(s)=w349:i32)
        n169 = case shown="1" w349 {
          tunnel: w351 -> [w355 w358]
          tunnel: [w354 w357] -> w348
          tunnel: ["Panel Hidden" ("Message") "Exit Prepare" ("Message")] -> w347
          frame 2, Default {
            n170 = Unbundle By Name(w355) -> ("Message"=w354:refnum<queue>)
          }
          frame 1 {
            n171 = Unbundle By Name(w358) -> ("Message"=w357:refnum<queue>)
          }
        }
        n172 = call "Queue In.vi"("First"=TRUE, "Message"=w347, "Queue In"=w348) -> ()  [unwired: 7 in, 2 out]
        n173 = event-data("Discard?"=TRUE ("放弃？")) -> ()  [unwired: 1 in, 1 out]
      }
      event "Data Source List": Value Change {
        n174 = event-data() -> ("CtlRef"=w363:refnum<vi>, "NewVal"=w361:string)  [unwired: 1 in]
        n175 = Unbundle By Name(w368) -> ("UI"=w367:refnum<queue>)
        n176 = property class="Tree (strict)"(reference=w363, "Active Item Tag"=w361) -> (reference out=w362:refnum<vi>, error out=w360:errorcluster)  [unwired: 1 in]
        n177 = invoke class="Tree (strict)" method="Navigate Tree.Get Path"(reference=w362, error in=w360, "tag"=w361) -> (error out=w359:errorcluster, "Navigate Tree:Get Path"=w366:string[])  [unwired: 1 in, 2 out]
        n178 = Array Size(array=w366) -> (size(s)=w365:i32)
        n179 = case shown="2" w365 {
          tunnel: [_ w370 w373] -> w364
          tunnel: w359 -> [_ w369 w372]
          frame 0, Default {
          }
          frame 1 {
            n180 = case shown="No Error" w369 {
              tunnel: ["Group Active" ("Message") _] -> w370
              frame No Error {
              }
              frame Error {
              }
            }
          }
          frame 2 {
            n181 = case shown="No Error" w372 {
              tunnel: ["Source Active" ("Message") _] -> w373
              frame No Error {
              }
              frame Error {
              }
            }
          }
        }
        n182 = call "Queue In.vi"("Message"=w364, "Queue In"=w367) -> ()  [unwired: 8 in, 2 out]
      }
      event "Data Source List": Shortcut Menu Selection (User) {
        n183 = event-data() -> ("ItemTag"=w375:string)  [unwired: 1 in]
        n184 = Unbundle By Name(w377) -> ("UI"=w376:refnum<queue>)
        n185 = call "Queue In.vi"("Message"=w375, "Queue In"=w376) -> ()  [unwired: 8 in, 2 out]
      }
      event "Data Source List": Shortcut Menu Activation? {
        n186 = event-data() -> ("MenuRef"=w380:refnum<k9>, "CtlRef"=w382:refnum<vi>)  [unwired: 1 in]
        n187 = property class="Tree (strict)"(reference=w382) -> (reference out=w383:refnum<vi>, error out=w384:errorcluster, "Active Item Tag"=w379:string, "Value"=w378:string)  [unwired: 1 in]
        n188 = case shown="\"eee\", Default" w378 {
          tunnel: w384 -> [w394 _]
          tunnel: w383 -> [w393 _]
          tunnel: [w391 _] -> w381
          tunnel: w380 -> [w390 w423]
          tunnel: w379 -> [w387 _]
          frame "eee", Default {
            n189 = invoke class="Tree (strict)" method="Navigate Tree.Get Path"(reference=w393, error in=w394, "tag"=w387) -> (reference out=w385:refnum<vi>, "Navigate Tree:Get Path"=w386:string[])  [unwired: 1 in, 2 out]
            n190 = Delete Menu Items(9:w390) -> (0:w388:errorcluster, 3:w389:refnum<k9>)  [unwired: 3 in]
            n191 = Array Size(array=w386) -> (size(s)=w392:i32)
            n192 = case shown="2" w392 {
              tunnel: [TRUE _ _] -> w391
              tunnel: w389 -> [_ w399 w410]
              tunnel: w388 -> [_ _ _]
              tunnel: w387 -> [_ w396 _]
              tunnel: w385 -> [_ _ w407]
              frame 0, Default {
              }
              frame 1 {
                n193 = case shown="\"eee\", Default" w396 {
                  tunnel: [string[] ["添加分组", "删除分组", "修改分组", "添加数据源"] ("项名称") string[] ["Source Group Add", "Source Group Delete", "Source Group Modify"] ("项名称")] -> w398
                  tunnel: [string[] ["Source Group Add", "Source Group Delete", "Source Group Modify", "Source Add"] ("项名称") string[] ["添加分组", "删除分组", "修改分组"] ("项名称")] -> w397
                  frame "eee", Default {
                  }
                  frame "" {
                  }
                }
                n194 = Insert Menu Items(7:w397, 8:w398, 9:w399) -> ()  [unwired: 3 in, 3 out]
              }
              frame 2 {
                n195 = for {
                  N: 7 -> [_]
                  tunnel: [w413] -> w405 mode=indexing
                  shift-right: [w411] -> _
                  shift-left: w407 -> [w415]
                  i -> [w414]
                  n196 = Increment(x=w414) -> (x+1=w412:i32)
                  n197 = property class="Tree (strict)"(reference=w415, "ActiveColNum"=w412) -> (reference out=w411:refnum<vi>, "Cell String"=w413:string)  [unwired: 1 in, 1 out]
                }
                n198 = Delete From Array(array=w405) -> (deleted portion=w404:string)  [unwired: 2 in, 1 out]
                n199 = case shown="\"True\"" w404 {
                  tunnel: [string[] ["添加数据源", "删除数据源", "修改数据源信息", "导入数据源", "导出数据源", "关闭数据源", "弹出数据源", "打开后面板", "打开配置目录"] ("项名称") string[] ["添加数据源", "删除数据源", "修改数据源信息", "导入数据源", "导出数据源", "启动数据源", "打开配置目录"] ("项名称")] -> w409
                  tunnel: [string[] ["Source Add", "Source Delete", "Source Modify", "Source Import", "Source Export", "Source Close", "Source Panel Show", "Source Show Block Dirgram", "Source Open Config Path"] ("项名称") string[] ["Source Add", "Source Delete", "Source Modify", "Source Import", "Source Export", "Source Launch", "Source Open Config Path"] ("项名称")] -> w408
                  frame "True" {
                  }
                  frame "False", Default {
                  }
                }
                n200 = Insert Menu Items(7:w408, 8:w409, 9:w410) -> ()  [unwired: 3 in, 3 out]
              }
            }
          }
          frame "" {
            n201 = Delete Menu Items(9:w423) -> (3:w422:refnum<k9>)  [unwired: 3 in, 1 out]
            n202 = Insert Menu Items(7:string[] ["Source Group Add"] ("项名称"), 8:string[] ["添加分组"] ("项名称"), 9:w422) -> ()  [unwired: 3 in, 3 out]
          }
        }
        n203 = event-data("Discard?"=w381) -> ()  [unwired: 1 in, 1 out]
      }
      event "Data Source List": Double Click {
        n204 = event-data() -> ("CtlRef"=w428:refnum<vi>)  [unwired: 1 in]
        n205 = property class="Tree (strict)"(reference=w428) -> (reference out=w430:refnum<vi>, error out=w432:errorcluster, "Active Item Tag"=w429:string)  [unwired: 1 in]
        n206 = invoke class="Tree (strict)" method="Navigate Tree.Get Path"(reference=w430, error in=w432, "tag"=w429) -> ("Navigate Tree:Get Path"=w431:string[])  [unwired: 1 in, 3 out]
        n207 = Array Size(array=w431) -> (size(s)=w427:i32)
        n208 = case shown="2" w427 {
          tunnel: [_ "Source Modify"] -> w424
          frame 0, Default {
          }
          frame 2 {
          }
        }
        n209 = Unbundle By Name(w426) -> ("UI"=w425:refnum<queue>)
        n210 = call "Queue In.vi"("Message"=w424, "Queue In"=w425) -> ()  [unwired: 8 in, 2 out]
      }
    }
  }
  n211 = while {
    tunnel: w10 -> [w443]
    tunnel: [w440] -> w8
    tunnel: [w439] -> w9
    shift-right: [w436] -> _
    shift-left: _ -> [w435]
    tunnel: w3 -> [w434]
    stop <- w447 stop-if-true
    n212 = call "Queue Out.vi"("Queue In"=w443) -> ("error out"=w446:errorcluster, "Data"=w444:variant, "Message"=w445:string, "Queue Out"=w442:refnum<queue>)  [unwired: 6 in, 1 out]
    n213 = case shown="\"Source Launch Check\"" w445 {
      selector: w445 -> [_ _ _ _ _ _ _ _ _ _ _ _ _ _ _ _ _ _ _ _ _ _ w1043 w1119 _ _ _ _]
      tunnel: w442 -> [w450 w460 w466 w486 w508 w520 w608 w624 w651 w668 w695 w722 w740 w758 w796 w841 w883 w907 w941 w960 w988 w1012 w1052 w1123 w1133 w1144 w1149 w1153]
      tunnel: w446 -> [w449 w459 w465 w485 w507 w519 w607 w623 w650 w667 w694 w721 w739 w757 w795 w840 w882 w906 w940 w959 w987 w1011 w1051 w1122 w1132 w1143 w1147 w1154]
      tunnel: [w450 w460 w466 w486 w508 w520 w608 w624 w651 w668 w695 w722 w740 w758 w796 w841 w883 w907 w941 w960 w988 w1012 w1052 w1123 w1133 w1144 w1148 w1153] -> w441
      tunnel: [w449 w459 w465 w485 w507 w519 w607 w623 w650 w667 w694 w721 w739 w757 w795 w840 w882 w906 w940 w959 w987 w1011 w1051 w1122 w1132 w1143 w1146 w1154] -> w438
      tunnel: [_ "Load Device Info,Refresh Source Tree" ("Message") "Source Launch Check" ("Message") _ "Source Launch Check" ("Message") _ _ w620 w648 w659 _ "Refresh Source Tree" ("Message") _ w746 w790 w830 w867 _ "Source Panel Insert" ("Message") _ "Refresh Source Tree" ("Message") _ w1040 _ _ _ "Quit" _] -> w437
      tunnel: [_ _ _ _ _ _ _ _ _ _ _ _ _ _ _ _ _ _ _ _ _ _ _ _ _ _ _ TRUE] -> w447
      tunnel: w444 -> [_ _ _ _ _ _ w605 _ _ _ _ _ _ _ _ _ _ _ _ _ _ _ _ _ _ _ _ _]
      tunnel: [w448 w457 w463 w469 w501 w511 w604 w618 w646 w660 w689 w720 w738 w747 w791 w831 w881 w896 w939 w955 w980 w1010 w1044 w1121 w1131 w1142 w1145 w1151] -> w436
      tunnel: w435 -> [w448 _ w464 w473 w503 w518 w606 w622 w645 w661 w690 w720 w737 w748 w792 w832 w881 w896 w938 w956 w981 w1010 w1045 w1121 w1131 w1142 w1145 w1151]
      tunnel: w434 -> [_ w454 _ _ _ _ _ _ _ _ _ _ _ _ _ _ _ _ _ _ _ _ _ _ _ _ _ _]
      frame "eee", Default {
      }
      frame "Init" {
        # "初始化，定义所有可能会用到的参数"
        n214 = control-ref of="Data Source List"() -> (w455:refnum<vi>)
        n215 = control-ref of="本VI"() -> (w453:refnum<vi>)
        n216 = Bundle By Name(cluster=T11 {"Queue"={"UI"=refnum, "Message"=refnum, "Data"=refnum, "Caller"=refnum, "Name"="000 Common", "Data Path"=path "", "Class Path"=path "", "SubPanel"=refnum, "Project Name"="", "MNT"="", "Title"="", "Data Source"=refnum, "Queue List"={}, "VI"=refnum, "UE"=refnum}, "Data Source List"=refnum, "SubPanel"=refnum, "Group"={"Group Title"=["Name", "Enable", "Path"], "Group Data"={"Name"="", "Enable"="", "Path"=""}, "Group Name"=[]}, "Source"={"Source Title"=["Device Name", "Device Model", "Device Driver", "IP Address", "Port", "Remark", "Enable", "Path"], "Source Data"={"Device Name"="", "Device Model"="", "Device Driver"="", "IP Address"="", "Port"="", "Remark"="", "Enable"="", "Path"=""}, "Source Name"=[]}, "All Panel"=[], "GroupInfo"={}, "Class"={}, "Version Path"=path "", "Source Launch?"=TRUE, "Launch"=TRUE}, "Data Source List"=w455, "Queue"=w454) -> (w457:T11)
        n217 = property class="VI"(reference=w453, "FP.State"=T4."Maximized" ("前面板窗口:状态")) -> ()  [unwired: 1 in, 2 out]
        n218 = property on="Show Info" class="Bool (strict)"("Val(Sgnl)"=TRUE ("值(信号)")) -> ()  [unwired: 2 in, 2 out]
      }
      frame "Module Launch" {
        n219 = Bundle By Name(cluster=w464, "Source Launch?"=TRUE) -> (w463:T11)
      }
      frame "Load Device Info" {
        # "加载当前框架下需要用到的驱动以及路径"
        n220 = call "006 System Gloabl Read&Write.vi"("RW"=enum16{"Read", "Write"}."Read") -> ("Config Path"=w467:path)  [unwired: 7 in, 3 out]
        n221 = Bundle By Name(cluster=w473, "Version Path"=w467) -> (w471:T11)
        n222 = Unbundle By Name(w471) -> ("Version Path"=w470:path)
        n223 = Build Path(base path=w470, name or relative path=path "Device.csv" ("名称或相对路径")) -> (appended path=w483:path)
        n224 = call-poly <vilib>:"Read Delimited Spreadsheet.vi"("file path (dialog if empty)"=w483, "delimiter (\\t)"="," ("delimiter (\\t)")) -> ("all rows"=w484:string[][])  [unwired: 8 in, 5 out]
        n225 = Unbundle By Name(w471) -> ("Class"=w472:T12)
        n226 = Current VI's Path() -> (path=w482:path)
        n227 = Build Path(base path=w482, name or relative path=path "../../../.." ("名称或相对路径")) -> (appended path=w481:path)
        n228 = Delete From Array(array=w484, length=1 ("长度"), index (row)=0 ("索引 (行)")) -> (array with subset deleted=w475:string[][])  [unwired: 1 in, 1 out]
        n229 = for {
          shift-right: [w499] -> w474
          shift-left: w472 -> [w494]
          tunnel: w481 -> [w498]
          tunnel: w475 -> [w497] mode=indexing
          n230 = Index Array(array=w497) -> (element #1=w496:string, element #2=w495:string, element #3=w488:string, element #4=w487:string, element #5=w491:string, element #6=w489:string)  [unwired: 6 in]
          n231 = Build Path(base path=w498, name or relative path=w491) -> (appended path=w490:path)
          n232 = Look In Map(map=w494, key=w487) -> (value=w493:T13)  [unwired: 1 in, 1 out]
          n233 = Bundle By Name(cluster=w493, "Device_Type"=w496, "Device_Manufacturer"=w495, "Driver"=w488, "Device_Model"=w487, "Class Path"=w490, "Defaule Config Path"=w489) -> (w492:T13)
          n234 = Insert Into Map(map in=w494, key=w487, value=w492) -> (map out=w499:T12)  [unwired: 2 out]
        }
        n235 = Bundle By Name(cluster=w471, "Class"=w474) -> (w469:T11)
      }
      frame "Refresh Source Tree" {
        # "刷新树形结构"
        n236 = Unbundle By Name(w503) -> ("Queue.Data Path"=w505:path, "Data Source List"=w504:refnum<vi>)
        n237 = call "Data Source Tree Refresh.vi"("Tree In"=w504, "Data Path"=w505) -> ("GroupInfo Out"=w502:T14, "Count"=→"Count":string)  [unwired: 7 in, 1 out]
        n238 = Bundle By Name(cluster=w503, "GroupInfo"=w502) -> (w501:T11)
      }
      frame "Source Launch Check" {
        # "启动核心，检查需要的驱动是否已经加载到内存中，若没有加载则加载"
        n239 = Unbundle By Name(w518) -> ("Queue.Data Path"=w517:path, "Queue.Project Name"=w514:string, "GroupInfo"=w513:T14)
        n240 = call <vilib>:"Check if File or Folder Exists.vi"("path"=w517) -> ("file or folder exists?"=w516:bool, "dup path"=w515:path)  [unwired: 8 in, 1 out]
        n241 = case shown="True" w516 {
          tunnel: w515 -> [_ w527]
          tunnel: w518 -> [w521 w525]
          tunnel: [w521 w525] -> w512
          tunnel: w514 -> [_ w526]
          tunnel: w513 -> [_ w524]
          tunnel: [_ w523] -> w510
          tunnel: [_ w522] -> w509
          frame False {
          }
          frame True {
            n242 = for {
              tunnel: w527 -> [w536]
              tunnel: w526 -> [w535]
              tunnel: w524 -> [w533] mode=indexing
              shift-right: [w530] -> _
              shift-left: w525 -> [w534]
              tunnel: [w529] -> w523 mode=concatenating
              tunnel: [w528] -> w522 mode=indexing
              # "遍历每一个模块分组"
              n243 = Unbundle By Name(w533) -> ("Group.Group.Path"=w531:string, "Group.Source"=w532:map{string, T10}, "Group.Group.Name"=w528:string)
              n244 = for {
                tunnel: w536 -> [w553]
                tunnel: w535 -> [w552]
                tunnel: w532 -> [w547] mode=indexing
                tunnel: w531 -> [w548]
                shift-right: [w539] -> w530
                shift-left: w534 -> [w540]
                tunnel: [w537] -> w529 mode=indexing
                # "遍历分组中每一个驱动"
                n245 = Unbundle By Name(w547) -> ("Data.Path"=w546:string, "Data.Device Name"=w545:string, "Data.Enable"=w541:string, "Data.Device Driver"=w538:string, "Data.Device Name"=w537:string)
                n246 = Build Path(base path=w553, name or relative path=w548) -> (appended path=w550:path)
                n247 = Build Path(base path=w550, name or relative path=w546) -> (appended path=w549:path)
                n248 = Unbundle By Name(w540) -> ("Queue.Queue List"=w544:map{string, refnum<queue>})
                n249 = Concatenate Strings(w552, "-" ("字符串"), w545) -> (w543:string)
                n250 = Look In Map(map=w544, key=w543) -> (key not found?=w542:bool)  [unwired: 1 in, 1 out]
                n251 = case shown="True" w542 {
                  tunnel: w549 -> [_ w561]
                  tunnel: w543 -> [_ w560]
                  tunnel: w541 -> [_ w559]
                  tunnel: w538 -> [_ w558]
                  tunnel: w540 -> [w554 w557]
                  tunnel: [w554 w556] -> w539
                  tunnel: w537 -> [_ w555]
                  frame False {
                  }
                  frame True {
                    # "检查该驱动是否已经加载到内存中"
                    n252 = case shown="\"True\"" w559 {
                      tunnel: w561 -> [_ w585]
                      tunnel: w560 -> [_ w580]
                      tunnel: w558 -> [_ w571]
                      tunnel: w557 -> [w562 w581]
                      tunnel: [w562 w570] -> w556
                      tunnel: w555 -> [_ w565]
                      frame Default {
                        # "已经加载到内存中即忽略"
                      }
                      frame "True" {
                        # "如果没有找到就加载空框架"
                        # "未加载到内存中根据相对路径加载"
                        n253 = case shown="\"WarningLog\"" w571 {
                          tunnel: w581 -> [w587 w589 w593 w597]
                          tunnel: [w587 w589 w593 w597] -> w570
                          tunnel: w580 -> [_ w588 w592 w596]
                          frame "eee", Default {
                            # "默认模块"
                          }
                          frame "WarningLog" {
                            # "特殊模块特殊处理"
                            n254 = Unbundle By Name(w589) -> ("Queue.Data"=w591:refnum<queue>)
                            n255 = call "Queue In.vi"("Data"=w588, "Message"="Log", "Queue In"=w591) -> ()  [unwired: 7 in, 2 out]
                          }
                          frame "LoadControl" {
                            # "特殊模块特殊处理"
                            n256 = Unbundle By Name(w593) -> ("Queue.Data"=w595:refnum<queue>)
                            n257 = call "Queue In.vi"("Data"=w592, "Message"="LoadControl", "Queue In"=w595) -> ()  [unwired: 7 in, 2 out]
                          }
                          frame "DataMonitor" {
                            # "特殊模块特殊处理"
                            n258 = Unbundle By Name(w597) -> ("Queue.Data"=w599:refnum<queue>)
                            n259 = call "Queue In.vi"("Data"=w596, "Message"="DataMonitor", "Queue In"=w599) -> ()  [unwired: 7 in, 2 out]
                          }
                        }
                        n260 = Unbundle By Name(w570) -> ("Class"=w579:T12)
                        n261 = vi-ref "功率计测试平台.vi"() -> (w577:refnum<vi>)
                        n262 = Format Date/Time String() -> (date/time string=w566:string)  [unwired: 3 in]
                        n263 = property class="VI"(reference=w577) -> ("Path"=w576:path)  [unwired: 1 in, 2 out]
                        n264 = Format Into String(format string="启动 \"%s\" %s" ("格式字符串"), w565, w566) -> (resulting string=w564:string)  [unwired: 2 in, 1 out]
                        n265 = Look In Map(map=w579, key=w571) -> (key not found?=w578:bool, value=w574:T13)  [unwired: 1 in]
                        n266 = Unbundle By Name(w570) -> ("Queue.Caller"=w569:refnum<queue>)
                        n267 = Unbundle By Name(w574) -> ("Class Path"=w573:path)
                        n268 = control-ref of="SubPanel"() -> (w583:refnum<vi>)
                        n269 = Unbundle By Name(w570) -> ("Source Launch?"=w572:bool, "Queue"=w582:T1)
                        n270 = Select(t=w576, s=w578, f=w573) -> (s? t:f=w575:path)
                        n271 = Bundle By Name(cluster=w582, "SubPanel"=w583, "Name"=w580, "Data Path"=w585, "Class Path"=w575) -> (w584:T1)
                        n272 = call "Queue In.vi"("Data"=w564, "Message"="Log", "Queue In"=w569) -> ()  [unwired: 7 in, 2 out]
                        n273 = Wait (ms)(milliseconds to wait=u32 100 ("等待时间（毫秒）")) -> ()  [unwired: 1 out]
                        n274 = case shown="True" w572 {
                          tunnel: w584 -> [_ w586]
                          frame False {
                          }
                          frame True {
                            n275 = call "000 Client Launch.vi"("Queue Ref"=w586) -> ()  [unwired: 10 in, 1 out]
                          }
                        }
                      }
                    }
                  }
                }
              }
            }
          }
        }
        n276 = Bundle By Name(cluster=w512, "Source.Source Name"=w510, "Group.Group Name"=w509) -> (w511:T11)
      }
      frame "Refresh Class Ref" {
        w601 = "Panel Name" ("Message")
        # "将所有子Alin的句柄名称发送至父Alin，父Alin可以根据队列名称对子Alin进行操作"
        n277 = in-place {
          in-place-border: w605 -> [w617]
          n278 = in-place-cluster #7(w606) -> ("Queue"=w616:T1)
          n279 = Variant To Data(type=w616, Variant=w617) -> (data=w615:T1)  [unwired: 1 in, 1 out]
          n280 = in-place-cluster #7("Queue"=w615) -> (w604:T11)
        }
        n281 = Unbundle By Name(w604) -> ("Queue.Queue List"=w602:map{string, refnum<queue>}, "Queue.Caller"=w603:refnum<queue>)
        n282 = for {
          tunnel: w602 -> [w614] mode=indexing
          tunnel: [w613] -> w600 mode=indexing
          n283 = Unbundle By Name(w614) -> ("Name"=w613:string)
        }
        n284 = call "Queue In.vi"("Data"=w600, "Message"=w601, "Queue In"=w603) -> ()  [unwired: 7 in, 2 out]
        n285 = for {
          tunnel: w602 -> [w612] mode=indexing
          tunnel: w601 -> [w610]
          tunnel: w600 -> [w609]
          n286 = Unbundle By Name(w612) -> ("Client Refer"=w611:refnum<queue>)
          n287 = call "Queue In.vi"("Data"=w609, "Message"=w610, "Queue In"=w611) -> ()  [unwired: 7 in, 2 out]
        }
      }
      frame "Source Group Add" {
        # "为驱动和模块添加分组"
        n288 = call "Data Source Add Group.vi"() -> ("OK？"=w621:bool, "Data Out"=w619:string[])  [unwired: 9 in, 1 out]
        n289 = case shown="True" w621 {
          tunnel: [_ w626] -> w620
          tunnel: w619 -> [_ w635]
          tunnel: w622 -> [w625 w628]
          tunnel: [w625 w629] -> w618
          frame False {
          }
          frame True {
            n290 = Array To Cluster(array=w635) -> (cluster=w634:T15)
            n291 = Bundle By Name(cluster=w628, "Group.Group Data"=w634) -> (w630:T11)
            n292 = Unbundle By Name(w630) -> ("Group.Group Name"=w632:string[], "Group.Group Data.Name"=w627:string)
            n293 = Search 1D Array(1D array=w632, element=w627) -> (index of element=w633:i32)  [unwired: 1 in]
            n294 = Less Than 0?(x=w633) -> (x < 0?=w631:bool)
            n295 = case shown="True" w631 {
              tunnel: w630 -> [_ w641]
              tunnel: w628 -> [w639 _]
              tunnel: [w639 w641] -> w629
              tunnel: w627 -> [w636 _]
              tunnel: [_ "Source Create Group Folder,Source Group Info Write"] -> w626
              frame False {
                n296 = Format Into String(format string="组名称”%s“已存在,请换个名称！" ("消息"), w636) -> (resulting string=w638:string)  [unwired: 2 in, 1 out]
                n297 = One Button Dialog(message=w638) -> ()  [unwired: 1 in, 1 out]
              }
              frame True {
              }
            }
          }
        }
      }
      frame "Source Group Modify" {
        # "修改分组信息"
        n298 = Unbundle By Name(w645) -> ("Group.Group Data"=w644:T9, "Group.Group Data.Path"=w642:string)
        n299 = Cluster To Array(cluster=w644) -> (array=w643:string[])
        n300 = call "Data Source Add Group.vi"("Data In"=w643) -> ("OK？"=w649:bool, "Data Out"=w647:string[])  [unwired: 8 in, 1 out]
        n301 = case shown="True" w649 {
          tunnel: [_ "Source Group Info Write"] -> w648
          tunnel: w647 -> [_ w655]
          tunnel: w645 -> [w652 w657]
          tunnel: [w652 w656] -> w646
          tunnel: w642 -> [_ w653]
          frame False {
          }
          frame True {
            n302 = Array To Cluster(array=w655) -> (cluster=w654:T15)
            n303 = Bundle By Name(cluster=w657, "Group.Group Data"=w654, "Group.Group Data.Path"=w653) -> (w656:T11)
          }
        }
      }
      frame "Source Group Delete" {
        # "删除分组以及该分组下面的所有数据源和模块"
        n304 = Unbundle By Name(w661) -> ("Group.Group Data.Path"=w662:string, "Data Source List"=w663:refnum<vi>)
        n305 = Format Into String(format string="确定删除分组 \"%s\"?" ("消息"), w662) -> (resulting string=w664:string)  [unwired: 2 in, 1 out]
        n306 = Two Button Dialog(message=w664) -> (T button?=w666:bool)  [unwired: 2 in]
        n307 = case shown="True" w666 {
          tunnel: w663 -> [_ w673]
          tunnel: w661 -> [w669 w675]
          tunnel: [w669 w675] -> w660
          tunnel: [_ "Refresh Source Tree"] -> w659
          frame False {
          }
          frame True {
            n308 = property class="Tree"(reference=w673, "ActiveColNum"=3 ("活动单元格:活动列数")) -> (error out=w672:errorcluster, "Cell String"=w671:string)  [unwired: 1 in, 1 out]
            n309 = case shown="No Error" w672 {
              tunnel: w675 -> [w677 _]
              tunnel: w671 -> [w676 _]
              frame No Error {
                n310 = case shown="\"eee\", Default" w676 {
                  selector: w676 -> [w682 _]
                  tunnel: w677 -> [w684 _]
                  frame "eee", Default {
                    n311 = Unbundle By Name(w684) -> ("Queue.Data Path"=w683:path)
                    n312 = Build Path(base path=w683, name or relative path=w682) -> (appended path=w681:path)
                    n313 = call <vilib>:"Check if File or Folder Exists.vi"("path"=w681) -> ("error out"=w678:errorcluster, "file or folder exists?"=w680:bool, "dup path"=w679:path)  [unwired: 8 in]
                    n314 = case shown="True" w680 {
                      tunnel: w679 -> [_ w687]
                      tunnel: w678 -> [_ w686]
                      frame False {
                      }
                      frame True {
                        n315 = Delete(path (use dialog)=w687, entire hierarchy (F)=TRUE ("整个层次结构(F)"), error in=w686) -> (error out=w685:errorcluster)  [unwired: 2 in, 2 out]
                        n316 = call <vilib>:"Clear Errors.vi"("error in (no error)"=w685) -> ()  [unwired: 5 in, 2 out]
                      }
                    }
                  }
                  frame "" {
                  }
                }
              }
              frame Error {
              }
            }
          }
        }
      }
      frame "Source Create Group Folder" {
        # "为分组添加不重复命名的文件夹"
        n317 = Unbundle By Name(w690) -> ("Queue.Data Path"=w693:path)
        n318 = call <vilib>:"Check if File or Folder Exists.vi"("path"=w693) -> ("file or folder exists?"=w692:bool, "dup path"=w691:path)  [unwired: 8 in, 1 out]
        n319 = case shown="True" w692 {
          tunnel: w691 -> [_ w709]
          tunnel: w690 -> [w696 w699]
          tunnel: [w696 w698] -> w689
          frame False {
          }
          frame True {
            n320 = List Folder(path=w709) -> (path out=w701:path, folder names=w708:string[])  [unwired: 3 in, 2 out]
            n321 = for {
              tunnel: w708 -> [w713] mode=indexing
              tunnel: [w710] -> w707 mode=indexing
              n322 = call <vilib>:"Delimited String to 1D String Array.vi"("delimiter"="_", "delimited string"=w713) -> ("string array"=w711:string[])  [unwired: 9 in]
              n323 = Index Array(array=w711) -> (element=w710:string)  [unwired: 1 in]
            }
            n324 = Fract/Exp String To Number(string=w707, default (0 dbl)=0 ("默认(0 DBL)")) -> (number=w705:i32[])  [unwired: 2 in, 1 out]
            n325 = Array Max & Min(array=w705) -> (max value=w703:i32)  [unwired: 3 out]
            n326 = Increment(x=w703) -> (x+1=w702:i32)
            n327 = Format Into String(format string="%03d_Group" ("格式字符串"), w702) -> (resulting string=w697:string)  [unwired: 2 in, 1 out]
            n328 = Build Path(base path=w701, name or relative path=w697) -> (appended path=w700:path)
            n329 = Bundle By Name(cluster=w699, "Group.Group Data.Path"=w697) -> (w698:T11)
            n330 = Create Folder(path (use dialog)=w700) -> ()  [unwired: 2 in, 3 out]
          }
        }
      }
      frame "Source Group Info Write" {
        # "分组信息写入"
        n331 = Unbundle By Name(w720) -> ("Queue.Data Path"=w718:path, "Group.Group Data.Path"=w719:string, "Group.Group Data"=w714:T9)
        n332 = call <vilib>:"Check if File or Folder Exists.vi"("path"=w718) -> ("file or folder exists?"=w717:bool, "dup path"=w716:path)  [unwired: 8 in, 1 out]
        n333 = case shown="True" w717 {
          tunnel: w719 -> [_ w727]
          tunnel: w716 -> [_ w729]
          tunnel: w714 -> [_ w728]
          frame False {
          }
          frame True {
            w724 = "info"
            n334 = Bundle By Name(cluster=w728, "Path"=w727) -> (w726:T9)
            n335 = Build Path(base path=w729, name or relative path=w727) -> (appended path=w732:path)
            n336 = Format Into String(format string="%s.ini" ("格式字符串"), w724) -> (resulting string=w730:string)  [unwired: 2 in, 1 out]
            n337 = Build Path(base path=w732, name or relative path=w730) -> (appended path=w723:path)
            n338 = call "Data Group RW.vi"("section"=w724, "Operate"=enum16{"Read", "Write"}."Write", "Source Path"=w723, "Group Type In"=w726) -> ()  [unwired: 4 in, 4 out]
          }
        }
      }
      frame "Group Active" {
        # "将活动分组加载到内存中"
        n339 = Unbundle By Name(w737) -> ("Group.Group Title"=w735:string[], "Data Source List"=w736:refnum<vi>)
        n340 = for {
          tunnel: [w743] -> w734 mode=indexing
          shift-right: [w741] -> _
          shift-left: w736 -> [w745]
          tunnel: w735 -> [_] mode=indexing
          i -> [w744]
          n341 = Increment(x=w744) -> (x+1=w742:i32)
          n342 = property class="Tree"(reference=w745, "ActiveColNum"=w742) -> (reference out=w741:refnum<vi>, "Cell String"=w743:string)  [unwired: 1 in, 1 out]
        }
        n343 = Array To Cluster(array=w734) -> (cluster=w733:T16)
        n344 = Bundle By Name(cluster=w737, "Group.Group Data"=w733) -> (w738:T11)
      }
      frame "Source Add" {
        # "添加数据源或者驱动，需要注意每一个模块或者驱动的命名不能重复，即使处于不同分组的模块名称也应该不同，如果有相同的程序会提示"
        n345 = Unbundle By Name(w748) -> ("Version Path"=w749:path, "Data Source List"=w756:refnum<vi>)
        n346 = property class="Tree"(reference=w756) -> (reference out=w754:refnum<vi>, error out=w752:errorcluster, "Active Item Tag"=w755:string)  [unwired: 1 in]
        n347 = invoke class="Tree" method="Navigate Tree.Get Path"(reference=w754, error in=w752, "tag"=w755) -> (error out=w750:errorcluster, "Navigate Tree:Get Path"=w753:string[])  [unwired: 1 in, 2 out]
        n348 = Array Size(array=w753) -> (size(s)=w751:i32)
        n349 = case shown="No Error" w750 {
          tunnel: w751 -> [w763 _]
          tunnel: w749 -> [w762 _]
          tunnel: w748 -> [w761 w788]
          tunnel: [w760 w788] -> w747
          tunnel: [w759 _] -> w746
          frame No Error {
            n350 = case shown="1, 2" w763 {
              tunnel: w762 -> [_ w765]
              tunnel: w761 -> [w764 w768]
              tunnel: [w764 w767] -> w760
              tunnel: [_ w766] -> w759
              frame 0, Default {
              }
              frame 1, 2 {
                n351 = call "DataSource Device Select.vi"("Version Path"=w765) -> ("OK？"=w770:bool, "Data Out"=w769:string[])  [unwired: 9 in]
                n352 = case shown="True" w770 {
                  tunnel: w769 -> [_ w781]
                  tunnel: w768 -> [w771 w774]
                  tunnel: [w771 w773] -> w767
                  tunnel: [_ w780] -> w766
                  frame False {
                  }
                  frame True {
                    n353 = Array To Cluster(array=w781) -> (cluster=w779:T17)
                    n354 = Bundle By Name(cluster=w774, "Source.Source Data"=w779) -> (w775:T11)
                    n355 = Unbundle By Name(w775) -> ("Source.Source Name"=w778:string[], "Source.Source Data.Device Name"=w772:string)
                    n356 = Search 1D Array(1D array=w778, element=w772) -> (index of element=w777:i32)  [unwired: 1 in]
                    n357 = Less Than 0?(x=w777) -> (x < 0?=w776:bool)
                    n358 = case shown="True" w776 {
                      tunnel: [_ "Source Create Folder,Source Config Load,Source Info Write"] -> w780
                      tunnel: w775 -> [_ w786]
                      tunnel: w774 -> [w785 _]
                      tunnel: [w785 w786] -> w773
                      tunnel: w772 -> [w782 _]
                      frame False {
                        n359 = Format Into String(format string="名称”%s“已存在,请换个名称！" ("消息"), w782) -> (resulting string=w783:string)  [unwired: 2 in, 1 out]
                        n360 = One Button Dialog(message=w783) -> ()  [unwired: 1 in, 1 out]
                      }
                      frame True {
                      }
                    }
                  }
                }
              }
            }
          }
          frame Error {
          }
        }
      }
      frame "Source Delete" {
        # "删除驱动或者模块以及其产生的所有配置信息"
        n361 = Unbundle By Name(w792) -> ("Source.Source Data.Path"=w793:string, "Data Source List"=w794:refnum<vi>, "Source.Source Data.Enable"=w789:string)
        n362 = case shown="\"eee\", Default" w789 {
          tunnel: w794 -> [w801 _]
          tunnel: w793 -> [w800 _]
          tunnel: w792 -> [w799 w828]
          tunnel: [w798 w828] -> w791
          tunnel: [w797 _] -> w790
          frame "eee", Default {
            n363 = Format Into String(format string="确定删除数据源 \"%s\"?" ("消息"), w800) -> (resulting string=w802:string)  [unwired: 2 in, 1 out]
            n364 = Two Button Dialog(message=w802) -> (T button?=w804:bool)  [unwired: 2 in]
            n365 = case shown="True" w804 {
              tunnel: w801 -> [_ w809]
              tunnel: w799 -> [w805 w811]
              tunnel: [w805 w811] -> w798
              tunnel: [_ "Refresh Source Tree"] -> w797
              frame False {
              }
              frame True {
                n366 = property class="Tree"(reference=w809, "ActiveColNum"=7 ("活动单元格:活动列数")) -> (error out=w808:errorcluster, "Cell String"=w806:string)  [unwired: 1 in, 1 out]
                n367 = case shown="No Error" w808 {
                  tunnel: w811 -> [w813 _]
                  tunnel: w806 -> [w812 _]
                  frame No Error {
                    n368 = case shown="\"eee\", Default" w812 {
                      tunnel: w813 -> [w822 _]
                      frame "eee", Default {
                        n369 = Unbundle By Name(w822) -> ("Queue.Data Path"=w821:path, "Group.Group Data.Path"=w817:string, "Source.Source Data.Path"=w815:string)
                        n370 = Build Path(base path=w821, name or relative path=w817) -> (appended path=w816:path)
                        n371 = Build Path(base path=w816, name or relative path=w815) -> (appended path=w814:path)
                        n372 = call <vilib>:"Check if File or Folder Exists.vi"("path"=w814) -> ("error out"=w818:errorcluster, "file or folder exists?"=w820:bool, "dup path"=w819:path)  [unwired: 8 in]
                        n373 = case shown="True" w820 {
                          tunnel: w819 -> [_ w825]
                          tunnel: w818 -> [_ w824]
                          frame False {
                          }
                          frame True {
                            n374 = Delete(path (use dialog)=w825, entire hierarchy (F)=TRUE ("整个层次结构(F)"), error in=w824) -> (error out=w823:errorcluster)  [unwired: 2 in, 2 out]
                            n375 = call <vilib>:"Clear Errors.vi"("error in (no error)"=w823) -> ()  [unwired: 5 in, 2 out]
                          }
                        }
                      }
                      frame "" {
                      }
                    }
                  }
                  frame Error {
                  }
                }
              }
            }
          }
          frame "True" {
            n376 = One Button Dialog(message="请先关闭数据源！" ("消息")) -> ()  [unwired: 1 in, 1 out]
          }
        }
      }
      frame "Source Modify" {
        # "修改模块信息"
        n377 = Unbundle By Name(w832) -> ("Data Source List"=w839:refnum<vi>, "Version Path"=w829:path)
        n378 = property class="Tree"(reference=w839) -> (reference out=w837:refnum<vi>, error out=w835:errorcluster, "Active Item Tag"=w838:string)  [unwired: 1 in]
        n379 = invoke class="Tree" method="Navigate Tree.Get Path"(reference=w837, error in=w835, "tag"=w838) -> (error out=w833:errorcluster, "Navigate Tree:Get Path"=w836:string[])  [unwired: 1 in, 2 out]
        n380 = Array Size(array=w836) -> (size(s)=w834:i32)
        n381 = case shown="No Error" w833 {
          tunnel: w834 -> [w846 _]
          tunnel: w832 -> [w845 w866]
          tunnel: [w844 w866] -> w831
          tunnel: [w843 _] -> w830
          tunnel: w829 -> [w842 _]
          frame No Error {
            n382 = case shown="1, 2" w846 {
              tunnel: w845 -> [w847 w853]
              tunnel: [w847 w855] -> w844
              tunnel: [_ w854] -> w843
              tunnel: w842 -> [_ w848]
              frame 0, Default {
              }
              frame 1, 2 {
                n383 = Unbundle By Name(w853) -> ("Source.Source Data"=w852:T10, "Source.Source Data.Path"=w849:string, "Source.Source Data.Enable"=w850:string)
                n384 = Cluster To Array(cluster=w852) -> (array=w851:string[])
                n385 = call "DataSource Device Select.vi"("Version Path"=w848, "Data In"=w851) -> ("OK？"=w857:bool, "Data Out"=w856:string[])  [unwired: 8 in]
                n386 = case shown="True" w857 {
                  tunnel: w856 -> [_ w863]
                  tunnel: w853 -> [w858 w865]
                  tunnel: [w858 w864] -> w855
                  tunnel: [_ "Source Info Write"] -> w854
                  tunnel: w850 -> [_ w860]
                  tunnel: w849 -> [_ w859]
                  frame False {
                  }
                  frame True {
                    n387 = Array To Cluster(array=w863) -> (cluster=w861:T17)
                    n388 = Bundle By Name(cluster=w865, "Source.Source Data"=w861, "Source.Source Data.Path"=w859, "Source.Source Data.Enable"=w860) -> (w864:T11)
                  }
                }
              }
            }
          }
          frame Error {
          }
        }
      }
      frame "Source Import" {
        # "为分组导入SDQ表"
        n389 = Unbundle By Name(w881) -> ("Queue.Data Path"=w880:path, "Group.Group Data.Path"=w879:string, "Source.Source Data.Path"=w877:string)
        n390 = Build Path(base path=w880, name or relative path=w879) -> (appended path=w878:path)
        n391 = Build Path(base path=w878, name or relative path=w877) -> (appended path=w876:path)
        n392 = Build Path(base path=w876, name or relative path=path "Data.csv" ("名称或相对路径")) -> (appended path=w872:path)
        n393 = call <vilib>:"Check if File or Folder Exists.vi"("path"=w872) -> ("file or folder exists?"=w871:bool, "dup path"=w870:path)  [unwired: 8 in, 1 out]
        n394 = case shown="True" w871 {
          tunnel: w870 -> [w884 w890]
          tunnel: [w884 w889] -> w869
          tunnel: [_ w885] -> w868
          frame False {
          }
          frame True {
            n395 = call-poly <vilib>:"Read Delimited Spreadsheet.vi"("file path (dialog if empty)"=w890, "delimiter (\\t)"="," ("delimiter (\\t)")) -> ("new file path (Not A Path if cancelled)"=w889:path, "all rows"=w888:string[][])  [unwired: 8 in, 4 out]
            n396 = Delete From Array(array=w888, length=1 ("长度"), index (row)=0 ("索引 (行)")) -> (array with subset deleted=w885:string[][])  [unwired: 1 in, 1 out]
          }
        }
        n397 = call "Data Source Import.vi"("Data In"=w868) -> ("OK?"=w874:bool, "Data"=w873:string[][])  [unwired: 9 in]
        n398 = case shown="True" w874 {
          tunnel: w869 -> [_ w895]
          tunnel: w873 -> [_ w894]
          tunnel: [_ "Data Load" ("Message")] -> w867
          frame False {
          }
          frame True {
            n399 = call-poly <vilib>:"Write Delimited Spreadsheet.vi"("file path (dialog if empty)"=w895, "2D data"=w894, "delimiter (\\t)"="," ("delimiter (\\t)")) -> ()  [unwired: 11 in, 2 out]
          }
        }
      }
      frame "Source Export" {
        # "导出SDQ表"
        n400 = Unbundle By Name(w896) -> ("Queue.Data Path"=w905:path, "Group.Group Data.Path"=w904:string, "Source.Source Data.Path"=w902:string)
        n401 = Build Path(base path=w905, name or relative path=w904) -> (appended path=w903:path)
        n402 = Build Path(base path=w903, name or relative path=w902) -> (appended path=w901:path)
        n403 = Build Path(base path=w901, name or relative path=path "Data.csv" ("名称或相对路径")) -> (appended path=w899:path)
        n404 = call <vilib>:"Check if File or Folder Exists.vi"("path"=w899) -> ("file or folder exists?"=w898:bool, "dup path"=w897:path)  [unwired: 8 in, 1 out]
        n405 = case shown="True" w898 {
          tunnel: w897 -> [_ w912]
          tunnel: w896 -> [_ w909]
          frame False {
          }
          frame True {
            n406 = Unbundle By Name(w909) -> ("Source.Source Data.Device Name"=w908:string)
            n407 = call "文件对话框"("default name"=w908, "pattern (all files)"="*.xlsx") -> ("selected path"=w914:path, "cancelled"=w913:bool, "error out"=w915:errorcluster)  [unwired: 10 in, 1 out]
            n408 = call-poly <vilib>:"Read Delimited Spreadsheet.vi"("file path (dialog if empty)"=w912, "delimiter (\\t)"="," ("delimiter (\\t)")) -> ("all rows"=w910:string[][])  [unwired: 8 in, 5 out]
            n409 = case shown="No Error" w915 {
              tunnel: w914 -> [w918 _]
              tunnel: w913 -> [w919 _]
              tunnel: w910 -> [w917 _]
              frame No Error {
                n410 = case shown="False" w919 {
                  tunnel: w918 -> [w921 _]
                  tunnel: w917 -> [w920 _]
                  frame False {
                    n411 = call "Excel Write.vi"("Write"=w920, "Path"=w921) -> ()  [unwired: 9 in, 1 out]
                  }
                  frame True {
                  }
                }
              }
              frame Error {
              }
            }
          }
        }
      }
      frame "Source Active" {
        # "将活动数据源信息加载到内存中"
        n412 = Unbundle By Name(w938) -> ("Source.Source Title"=w929:string[], "Data Source List"=w932:refnum<vi>, "Group.Group Title"=w923:string[])
        n413 = for {
          tunnel: [w949] -> w925 mode=indexing
          shift-right: [w947] -> w937
          shift-left: w932 -> [w951]
          tunnel: w929 -> [_] mode=indexing
          i -> [w950]
          n414 = Increment(x=w950) -> (x+1=w948:i32)
          n415 = property class="Tree"(reference=w951, "ActiveColNum"=w948) -> (reference out=w947:refnum<vi>, "Cell String"=w949:string)  [unwired: 1 in, 1 out]
        }
        n416 = property class="Tree"(reference=w932) -> ("Value"=w931:variant)  [unwired: 1 in, 2 out]
        n417 = Variant To Data(type="" ("Data Source List"), Variant=w931) -> (data=w924:string)  [unwired: 1 in, 1 out]
        n418 = invoke class="Tree" method="Navigate Tree.Get Parent"(reference=w937, "tag"=w924) -> (reference out=w936:refnum<vi>, "Navigate Tree:Get Parent"=w935:string)  [unwired: 2 in, 2 out]
        n419 = property class="Tree"(reference=w936, "Active Item Tag"=w935) -> (reference out=w934:refnum<vi>)  [unwired: 1 in, 1 out]
        n420 = for {
          tunnel: [w944] -> w928 mode=indexing
          shift-right: [w942] -> w933
          shift-left: w934 -> [w946]
          tunnel: w923 -> [_] mode=indexing
          i -> [w945]
          n421 = Increment(x=w945) -> (x+1=w943:i32)
          n422 = property class="Tree"(reference=w946, "ActiveColNum"=w943) -> (reference out=w942:refnum<vi>, "Cell String"=w944:string)  [unwired: 1 in, 1 out]
        }
        n423 = Array To Cluster(array=w925) -> (cluster=w926:T18)
        n424 = Array To Cluster(array=w928) -> (cluster=w927:T16)
        n425 = property class="Tree"(reference=w933, "Active Item Tag"=w924) -> ()  [unwired: 1 in, 2 out]
        n426 = Bundle By Name(cluster=w938, "Source.Source Data"=w926, "Group.Group Data"=w927) -> (w939:T11)
      }
      frame "Source Create Folder" {
        # "添加数据源的文件夹，该分组下的文件夹命名自增不重复"
        n427 = Unbundle By Name(w956) -> ("Queue.Data Path"=w954:path, "Group.Group Data.Path"=w953:string)
        n428 = Build Path(base path=w954, name or relative path=w953) -> (appended path=w952:path)
        n429 = call <vilib>:"Check if File or Folder Exists.vi"("path"=w952) -> ("file or folder exists?"=w958:bool, "dup path"=w957:path)  [unwired: 8 in, 1 out]
        n430 = case shown="True" w958 {
          tunnel: w957 -> [_ w974]
          tunnel: w956 -> [w961 w964]
          tunnel: [w961 w963] -> w955
          frame False {
          }
          frame True {
            n431 = List Folder(path=w974) -> (path out=w966:path, folder names=w973:string[])  [unwired: 3 in, 2 out]
            n432 = for {
              tunnel: w973 -> [w978] mode=indexing
              tunnel: [w975] -> w972 mode=indexing
              n433 = call <vilib>:"Delimited String to 1D String Array.vi"("delimiter"="_", "delimited string"=w978) -> ("string array"=w976:string[])  [unwired: 9 in]
              n434 = Index Array(array=w976) -> (element=w975:string)  [unwired: 1 in]
            }
            n435 = Fract/Exp String To Number(string=w972, default (0 dbl)=0 ("默认(0 DBL)")) -> (number=w970:i32[])  [unwired: 2 in, 1 out]
            n436 = Array Max & Min(array=w970) -> (max value=w968:i32)  [unwired: 3 out]
            n437 = Increment(x=w968) -> (x+1=w967:i32)
            n438 = Format Into String(format string="%03d_Source" ("格式字符串"), w967) -> (resulting string=w962:string)  [unwired: 2 in, 1 out]
            n439 = Build Path(base path=w966, name or relative path=w962) -> (appended path=w965:path)
            n440 = Bundle By Name(cluster=w964, "Source.Source Data.Path"=w962) -> (w963:T11)
            n441 = Create Folder(path (use dialog)=w965) -> ()  [unwired: 2 in, 3 out]
          }
        }
      }
      frame "Source Info Write" {
        # "写入数据源信息"
        n442 = Unbundle By Name(w981) -> ("Queue.Data Path"=w979:path, "Group.Group Data.Path"=w986:string, "Source.Source Data.Path"=w982:string)
        n443 = call <vilib>:"Check if File or Folder Exists.vi"("path"=w979) -> ("file or folder exists?"=w985:bool, "dup path"=w984:path)  [unwired: 8 in, 1 out]
        n444 = case shown="True" w985 {
          tunnel: w986 -> [_ w998]
          tunnel: w984 -> [_ w999]
          tunnel: w982 -> [_ w995]
          tunnel: w981 -> [w989 w992]
          tunnel: [w989 w992] -> w980
          frame False {
          }
          frame True {
            w990 = "info"
            n445 = Build Path(base path=w999, name or relative path=w998) -> (appended path=w997:path)
            n446 = Build Path(base path=w997, name or relative path=w995) -> (appended path=w996:path)
            n447 = Format Into String(format string="%s.ini" ("格式字符串"), w990) -> (resulting string=w1000:string)  [unwired: 2 in, 1 out]
            n448 = Build Path(base path=w996, name or relative path=w1000) -> (appended path=w994:path)
            n449 = Unbundle By Name(w992) -> ("Source.Source Data"=w991:T10)
            n450 = call "Data Source RW.vi"("section"=w990, "Operate"=enum16{"Read", "Write"}."Write", "Source Path"=w994, "Data Type In"=w991) -> ()  [unwired: 4 in, 4 out]
          }
        }
      }
      frame "Source Config Load" {
        # "从默认路径下面加载改数据源的配置信息"
        n451 = Unbundle By Name(w1010) -> ("Queue.Data Path"=w1004:path, "Group.Group Data.Path"=w1003:string, "Source.Source Data.Path"=w1002:string, "Version Path"=w1005:path, "Class"=w1009:T12, "Source.Source Data.Device Driver"=w1008:string)
        n452 = Look In Map(map=w1009, key=w1008) -> (value=w1007:T13)  [unwired: 1 in, 1 out]
        n453 = Unbundle By Name(w1007) -> ("Defaule Config Path"=w1006:string)
        n454 = case shown="Default" w1006 {
          selector: w1006 -> [w1019 _]
          tunnel: w1005 -> [w1020 _]
          tunnel: w1004 -> [w1015 _]
          tunnel: w1003 -> [w1014 _]
          tunnel: w1002 -> [w1013 _]
          frame Default {
            n455 = Build Path(base path=w1020, name or relative path=w1019) -> (appended path=w1018:path)
            n456 = call <vilib>:"Check if File or Folder Exists.vi"("path"=w1018) -> ("file or folder exists?"=w1017:bool, "dup path"=w1016:path)  [unwired: 8 in, 1 out]
            n457 = case shown="True" w1017 {
              tunnel: w1016 -> [_ w1028]
              tunnel: w1015 -> [_ w1030]
              tunnel: w1014 -> [_ w1029]
              tunnel: w1013 -> [_ w1022]
              frame False {
              }
              frame True {
                n458 = List Folder(path=w1028) -> (path out=w1024:path, filenames=w1027:string[], folder names=w1026:string[])  [unwired: 3 in, 1 out]
                n459 = Build Path(base path=w1030, name or relative path=w1029) -> (appended path=w1023:path)
                n460 = Build Array (concatenate)(w1027, w1026) -> (w1025:string[])
                n461 = Build Path(base path=w1023, name or relative path=w1022) -> (appended path=w1021:path)
                n462 = for {
                  tunnel: w1025 -> [w1032] mode=indexing
                  tunnel: w1024 -> [w1033]
                  tunnel: w1021 -> [w1031]
                  n463 = case shown="\"info.ini\"" w1032 {
                    selector: w1032 -> [w1038 _]
                    tunnel: w1033 -> [w1039 _]
                    tunnel: w1031 -> [w1034 _]
                    frame Default {
                      n464 = Build Path(base path=w1039, name or relative path=w1038) -> (appended path=w1035:path)
                      n465 = Copy(9:TRUE ("覆盖(F)"), 10:w1034, 11:w1035) -> (0:w1036:errorcluster)  [unwired: 2 in, 2 out]
                      n466 = call <vilib>:"Clear Errors.vi"("error in (no error)"=w1036) -> ()  [unwired: 5 in, 2 out]
                    }
                    frame "info.ini" {
                    }
                  }
                }
              }
            }
          }
          frame "" {
          }
        }
      }
      frame "Data Load", "Source Close", "Source Launch", "Source Open Config Path", "Source Panel Insert", "Source Panel Show", "Source Show Block Dirgram" {
        # "从内存当中找到需要操作的数据源并且执行相关的操作"
        n467 = Unbundle By Name(w1045) -> ("Queue.Data Path"=w1049:path, "Group.Group Data.Path"=w1050:string, "Source.Source Data.Path"=w1046:string, "Queue.Project Name"=w1042:string, "Source.Source Data.Device Name"=w1041:string)
        n468 = call <vilib>:"Check if File or Folder Exists.vi"("path"=w1049) -> ("file or folder exists?"=w1048:bool, "dup path"=w1047:path)  [unwired: 8 in, 1 out]
        n469 = case shown="True" w1048 {
          tunnel: w1050 -> [_ w1066]
          tunnel: w1047 -> [_ w1067]
          tunnel: w1046 -> [_ w1065]
          tunnel: w1045 -> [w1053 w1060]
          tunnel: [w1053 w1060] -> w1044
          tunnel: w1043 -> [_ w1057]
          tunnel: w1042 -> [_ w1063]
          tunnel: w1041 -> [_ w1062]
          tunnel: [_ w1055] -> w1040
          frame False {
          }
          frame True {
            w1068 = "info"
            n470 = Build Path(base path=w1067, name or relative path=w1066) -> (appended path=w1058:path)
            n471 = Concatenate Strings(w1063, "-" ("字符串"), w1062) -> (w1059:string)
            n472 = Build Path(base path=w1058, name or relative path=w1065) -> (appended path=w1056:path)
            n473 = Format Into String(format string="%s.ini" ("格式字符串"), w1068) -> (resulting string=w1069:string)  [unwired: 2 in, 1 out]
            n474 = Build Path(base path=w1056, name or relative path=w1069) -> (appended path=w1054:path)
            n475 = case shown="\"Source Show Block Dirgram\"" w1057 {
              tunnel: ["True" "False" _ _ _ _ _] -> w1064
              tunnel: w1060 -> [_ w1086 w1093 w1099 w1105 w1112 _]
              tunnel: w1059 -> [_ w1084 w1091 w1097 w1103 w1110 _]
              tunnel: w1056 -> [_ _ _ _ _ _ _]
              tunnel: w1054 -> [_ _ _ _ _ _ w1116]
              frame "Source Launch", Default {
                # "启动数据源"
              }
              frame "Source Close" {
                # "将数据源从内存中移除"
                n476 = Unbundle By Name(w1086) -> ("Queue.Queue List"=w1085:map{string, refnum<queue>})
                n477 = Look In Map(map=w1085, key=w1084) -> (value=w1083:refnum<queue>)  [unwired: 1 in, 1 out]
                n478 = call "Queue In.vi"("First"=TRUE, "Message"="Exit Prepare", "Queue In"=w1083) -> ()  [unwired: 7 in, 2 out]
              }
              frame "Source Panel Show" {
                # "打开数据源前面板"
                n479 = Unbundle By Name(w1093) -> ("Queue.Queue List"=w1092:map{string, refnum<queue>})
                n480 = Look In Map(map=w1092, key=w1091) -> (value=w1090:refnum<queue>)  [unwired: 1 in, 1 out]
                n481 = call "Queue In.vi"("First"=TRUE, "Message"="Panel Show", "Queue In"=w1090) -> ()  [unwired: 7 in, 2 out]
              }
              frame "Source Show Block Dirgram" {
                # "打开数据源后面板"
                n482 = Unbundle By Name(w1099) -> ("Queue.Queue List"=w1098:map{string, refnum<queue>})
                n483 = Look In Map(map=w1098, key=w1097) -> (value=w1096:refnum<queue>)  [unwired: 1 in, 1 out]
                n484 = call "Queue In.vi"("First"=TRUE, "Message"="Show Block Dirgram", "Queue In"=w1096) -> ()  [unwired: 7 in, 2 out]
              }
              frame "Data Load" {
                # "加载数据"
                n485 = Unbundle By Name(w1105) -> ("Queue.Queue List"=w1104:map{string, refnum<queue>})
                n486 = Look In Map(map=w1104, key=w1103) -> (value=w1102:refnum<queue>)  [unwired: 1 in, 1 out]
                n487 = call "Queue In.vi"("First"=TRUE, "Message"="Data Load", "Queue In"=w1102) -> ()  [unwired: 7 in, 2 out]
              }
              frame "Source Panel Insert" {
                # "插入子面板"
                n488 = Unbundle By Name(w1112) -> ("Queue.Queue List"=w1111:map{string, refnum<queue>})
                n489 = control-ref of="SubPanel"() -> (w1107:refnum<vi>)
                n490 = Look In Map(map=w1111, key=w1110) -> (value=w1109:refnum<queue>)  [unwired: 1 in, 1 out]
                n491 = call "Queue In.vi"("First"=TRUE, "Data"=w1107, "Message"="SubPanel Change", "Queue In"=w1109) -> ()  [unwired: 6 in, 2 out]
              }
              frame "Source Open Config Path" {
                # "打开数据源的配置目录"
                n492 = call <vilib>:"Check if File or Folder Exists.vi"("path"=w1116) -> ("error out"=w1113:errorcluster, "file or folder exists?"=w1114:bool, "dup path"=w1115:path)  [unwired: 8 in]
                n493 = case shown="True" w1114 {
                  tunnel: w1115 -> [_ w1118]
                  tunnel: w1113 -> [_ w1117]
                  frame False {
                  }
                  frame True {
                    n494 = call <vilib>:"Show in File System.vi"("error in (no error)"=w1117, "file or directory path"=w1118) -> ()  [unwired: 9 in, 1 out]
                  }
                }
              }
            }
            n495 = case shown="\"eee\", Default" w1064 {
              selector: w1064 -> [w1072 _]
              tunnel: w1054 -> [w1079 _]
              tunnel: w1068 -> [w1078 _]
              tunnel: ["Refresh Source Tree" ("Message") _] -> w1055
              frame "eee", Default {
                n496 = call <vilib>:"Open Config Data.vi"("configuration file path"=w1079) -> ("error out"=w1075:errorcluster, "refnum"=w1077:T19)  [unwired: 8 in, 1 out]
                n497 = call-poly <vilib>:"Write Key.vi"("section"=w1078, "error in (no error)"=w1075, "value"=w1072, "key"="Enable", "refnum"=w1077) -> ("error out"=w1074:errorcluster, "refnum out"=w1076:T19)  [unwired: 4 in, 1 out]
                n498 = call <vilib>:"Close Config Data.vi"("error in (no error)"=w1074, "refnum"=w1076) -> ()  [unwired: 8 in, 2 out]
              }
              frame "" {
              }
            }
          }
        }
      }
      frame "Panel Show" {
        n499 = Unbundle By Name(w1121) -> ("Queue.Message"=w1120:refnum<queue>)
        n500 = call "Queue In.vi"("Message"=w1119, "Queue In"=w1120) -> ()  [unwired: 8 in, 2 out]
      }
      frame "FCTS DAQ" {
        n501 = property class="App"() -> ("App.Kind"=w1126:T20)  [unwired: 2 in, 2 out]
        n502 = case shown="\"invalid app kind\", Default" w1126 {
          tunnel: [path "Modules/002 Driver/004 Web DAQ SDK/Timedose.DAQ.Client.Test.exe" ("名称或相对路径") path "data/Timedose.DAQ.Client.Test.exe" ("名称或相对路径")] -> w1128
          frame "invalid app kind", Default {
          }
          frame "Run Time System" {
          }
        }
        n503 = call <vilib>:"Application Directory.vi"() -> ("Application Directory"=w1127:path)
        n504 = Build Path(base path=w1127, name or relative path=w1128) -> (appended path=w1129:path)
        n505 = Path To String(path=w1129) -> (string=w1130:string)
        n506 = call <vilib>:"System Exec.vi"("wait until completion? (T)"=FALSE, "command line"=w1130) -> ("error out"=w1124:errorcluster)  [unwired: 6 in, 3 out]
        n507 = call <vilib>:"Clear Errors.vi"("error in (no error)"=w1124) -> ()  [unwired: 5 in, 2 out]
      }
      frame "CAN Convert" {
        n508 = call <vilib>:"Application Directory.vi"() -> ("Application Directory"=w1138:path)
        n509 = Build Path(base path=w1138, name or relative path=path "Data/车辆技术DBC.exe" ("名称或相对路径")) -> (appended path=w1140:path)
        n510 = Path To String(path=w1140) -> (string=w1141:string)
        n511 = call <vilib>:"System Exec.vi"("wait until completion? (T)"=FALSE, "command line"=w1141) -> ("error out"=w1136:errorcluster)  [unwired: 6 in, 3 out]
        n512 = call <vilib>:"Clear Errors.vi"("error in (no error)"=w1136) -> ()  [unwired: 5 in, 2 out]
      }
      frame "Exit" {
        n513 = call "Queue Clear.vi"("error in (no error)"=w1147, "Queue In"=w1149) -> ("error out"=w1146:errorcluster, "Queue Out"=w1148:refnum<queue>)  [unwired: 8 in]
      }
      frame "Quit" {
      }
    }
    n514 = call "Queue In.vi"("error in (no error)"=w438, "Message"=w437, "Queue In"=w441) -> ("error out"=w439:errorcluster, "Queue Out"=w440:refnum<queue>)  [unwired: 7 in]
  }
  n515 = call "000 Driver Message.vi"("Queue In"=w3) -> ("error out"=w20:errorcluster)  [unwired: 8 in, 2 out]
  n516 = call "Queue Release.vi"("error in (no error)"=w17, "Queue In"=w16) -> ("error out"=w19:errorcluster)  [unwired: 9 in]
  n517 = call "Queue Release.vi"("error in (no error)"=w9, "Queue In"=w8) -> ("error out"=w12:errorcluster)  [unwired: 9 in]
  n518 = Unregister For Events(event registration refnum=w6) -> (error out=w7:errorcluster)  [unwired: 1 in]
  n519 = Destroy User Event(user event=w4, error in=w7) -> (error out=w11:errorcluster)
  n520 = Call Chain() -> (call chain=w14:string[])
  n521 = Merge Errors(w11, w12, w20, w19) -> (w13:errorcluster)
  n522 = Array Size(array=w14) -> (size(s)=w15:i32)
  n523 = case shown="2.." w15 {
    tunnel: w13 -> [_ w1155]
    frame 0, Default {
    }
    frame 2.. {
      n524 = invoke class="VI" method="FP.Close"(error in=w1155) -> ()  [unwired: 2 in, 3 out]
    }
  }
